vi "Main.vi"() -> ()   [LabVIEW 2013]
uses:
  <vilib>/Utility/miscctls.llb/LVFontTypeDef.ctl
panel:
  in  "SetCurrent":dbl min=0.0 max=72.0 step=0.1 format="%#.1g"
  in  "SetVoltage":dbl min=0.0 max=30.0 step=0.1 format="%#.1g"
  in  "SetCurrentB":bool
  in  "SetVoltageB":bool
  in  "Comm. current %":dbl=0.5 caption="%" min=0.0 max=100.0 step=0.5
  in  "Common curr. dec":bool
  in  "Common curr. inc":bool
  out "Дата":string
  out "Время":string
  in  "SetCurrentAll":bool
  in  "SetVoltageAll":bool
  in  "ConnectAll":bool
  in  "DisconnectAll":bool
  in  "Set Output ON All":bool caption="ВЫХОДЫ ИСТОЧНИКОВ"
  in  "Comm. voltage %":dbl caption="%" min=0.0 max=100.0 step=0.5
  in  "Common volt. dec":bool
  in  "Common volt. inc":bool
  in  "ReadFromFile":bool
  in  "WriteToFile":bool
  in  "SetOutputOffB":bool
  in  "SetOutputOnB":bool
  in  "ConnectChannel":bool
  in  "DisconnectChannel":bool
  in  "Имя":string="55"
  in  "DeleteChannel":bool
  in  "IP":string="172.16.21.19"
  in  "AddChannel":bool
  out "CURRENTSET":dbl[](array[numeric])
  in  "CurrentModulationOn":bool
  in  "Amp":dbl
  in  "CurrentModulationB":bool
  out "NAME":string[](array[string])
  out "ADRESS":string[](array[string])
  out "VIRef":refnum<vi>[](array[refnum])
  in  "Quit":bool
  in  "List of channels":i32(listbox)
  # "ВСЕ ИСТОЧНИКИ"
  # "1 ИСТОЧНИК"
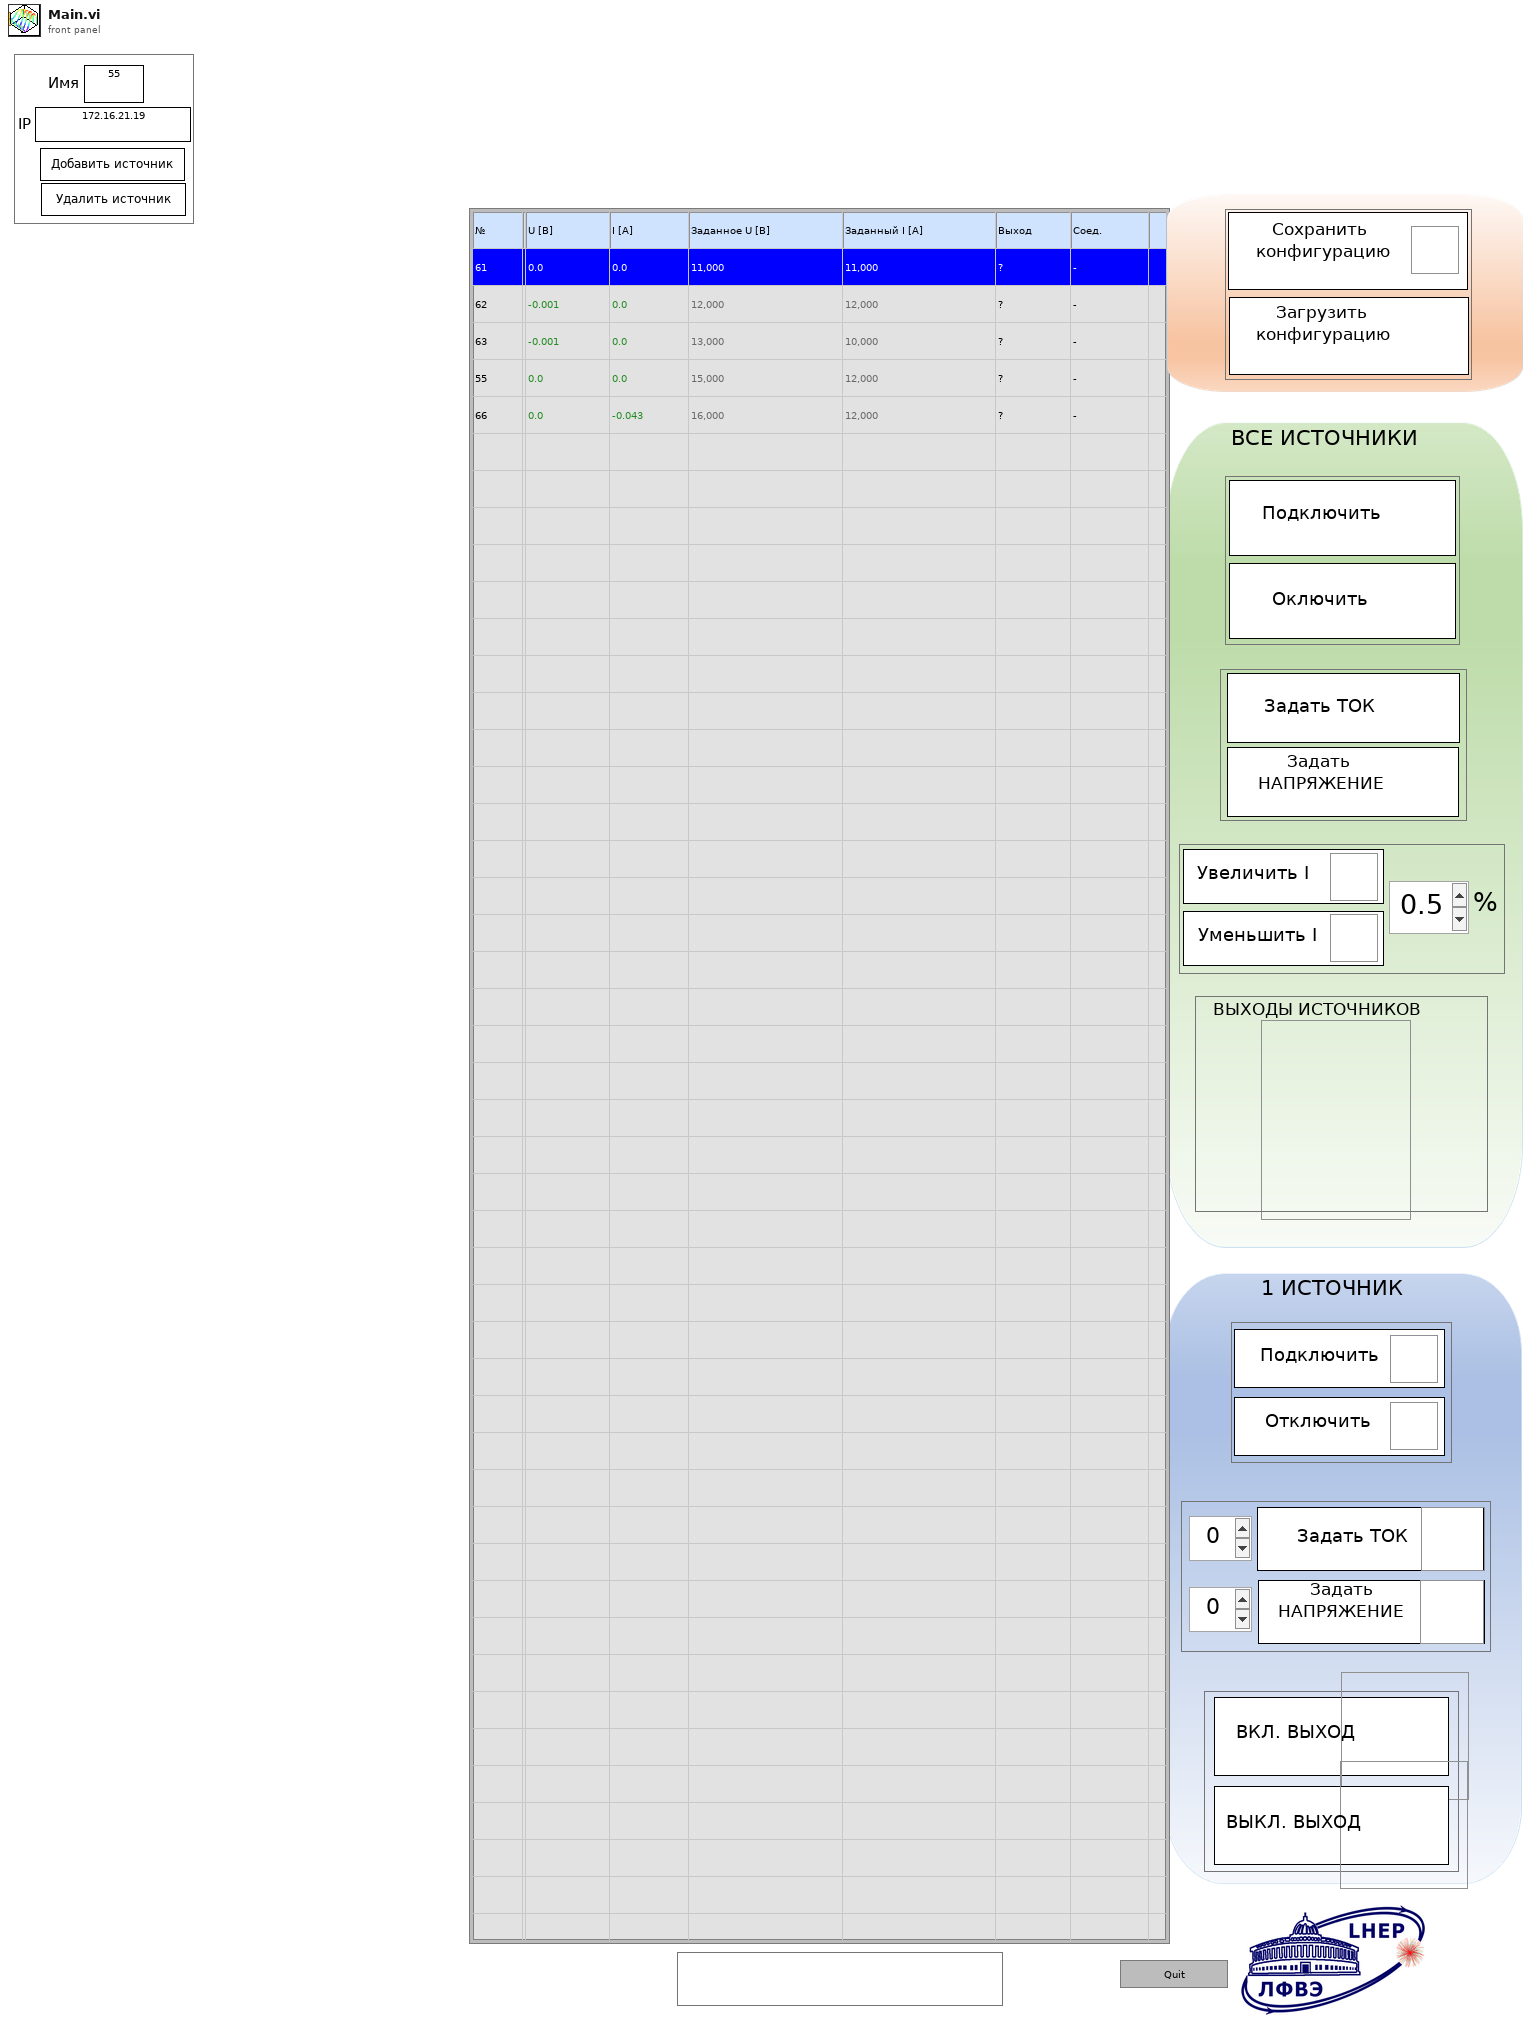
[diagram p1: front panel]
types:
  T1 = typedef "LVFontTypeDef.ctl" = cluster{"Font Name":string, "Size":u16, "Bold":bool, "Italic":bool, "Underline":bool, "Strikeout":bool, "Color":u32}
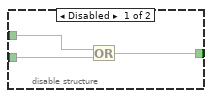
[diagram p3: hidden frame]
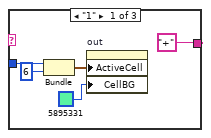
[diagram p4: hidden frame]
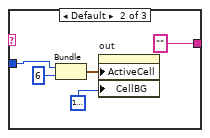
[diagram p5: hidden frame]
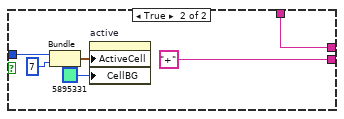
[diagram p6: hidden frame]
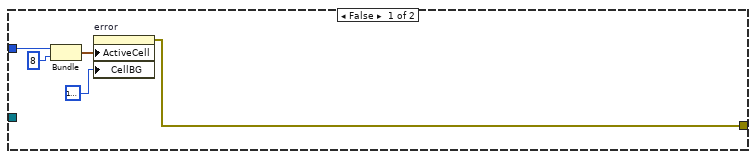
[diagram p7: hidden frame]
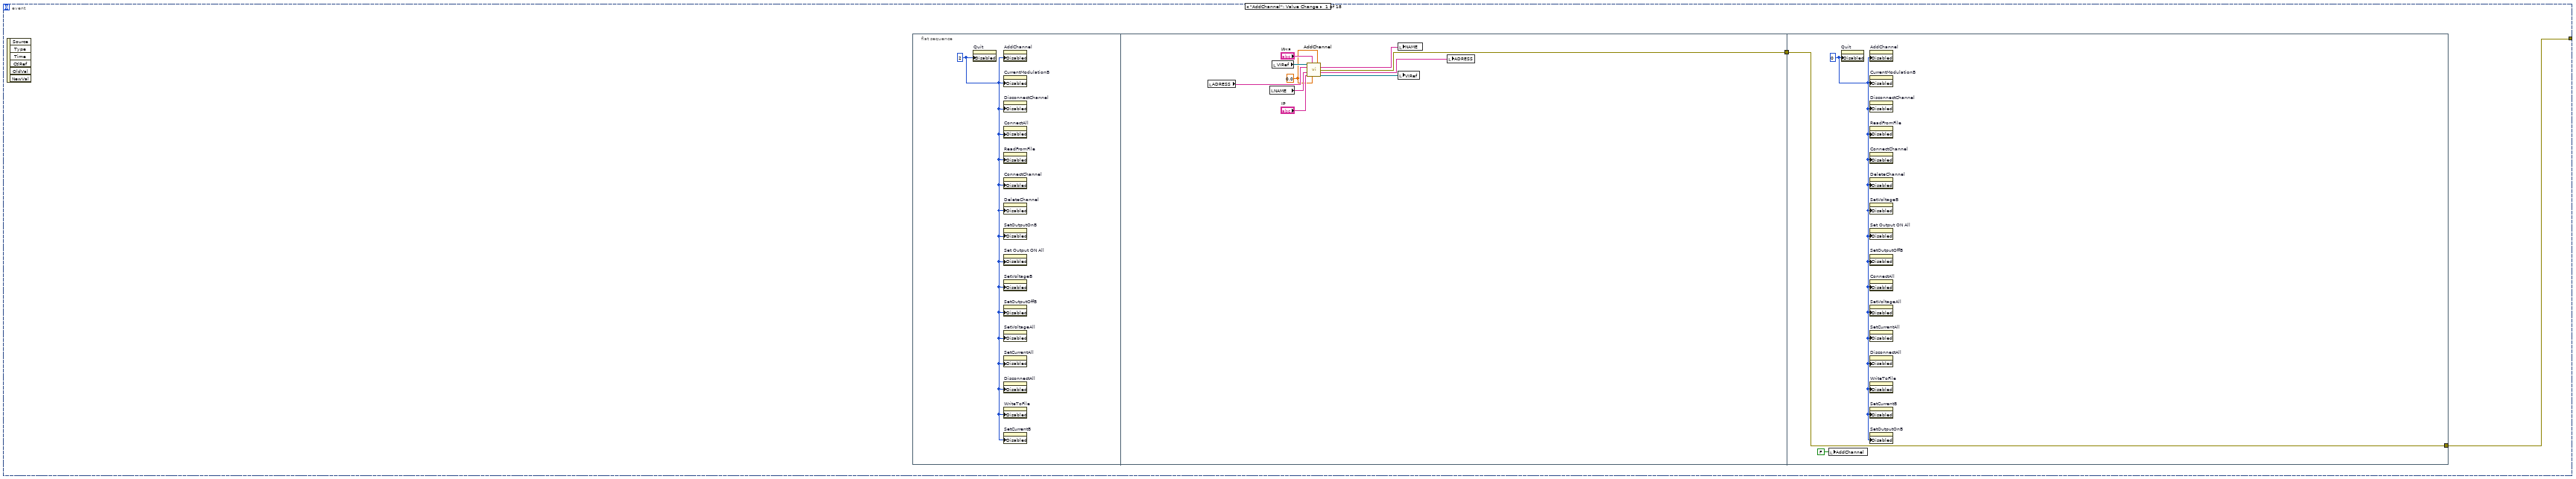
[diagram p8: hidden frame]
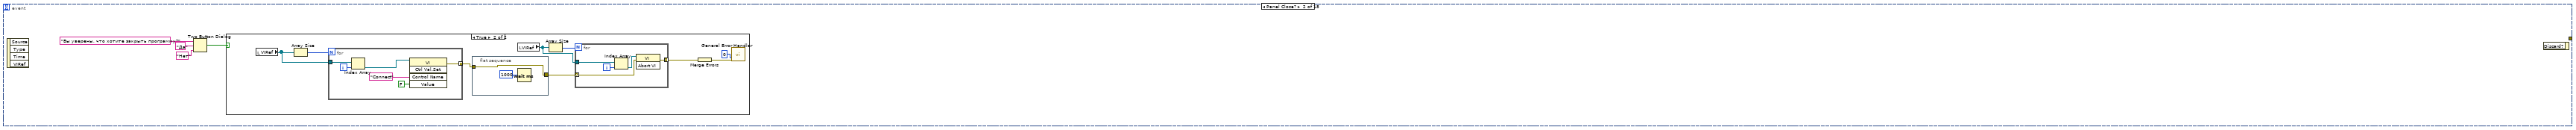
[diagram p9: hidden frame]
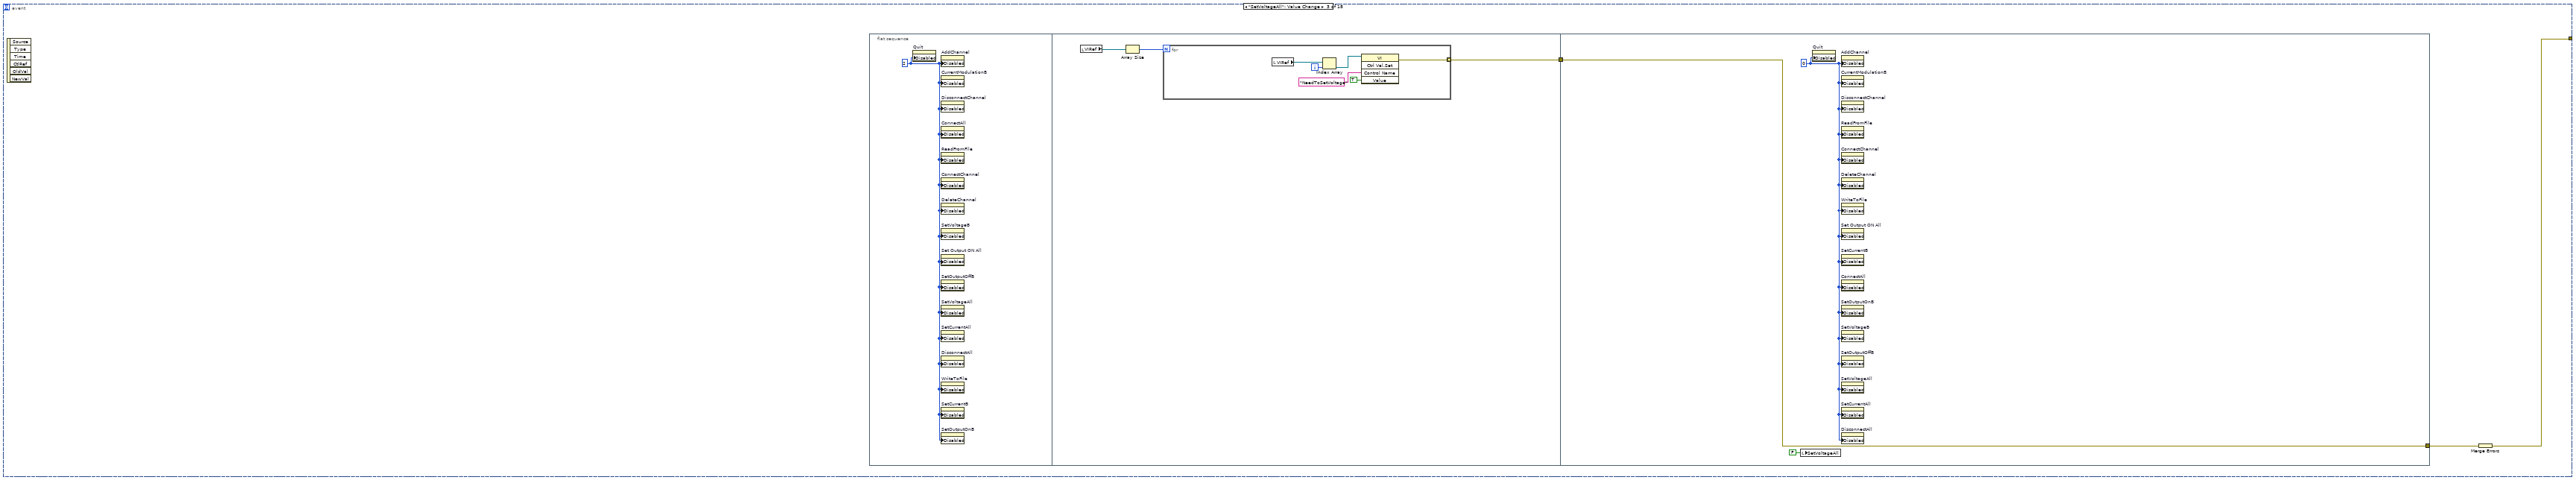
[diagram p11: hidden frame]
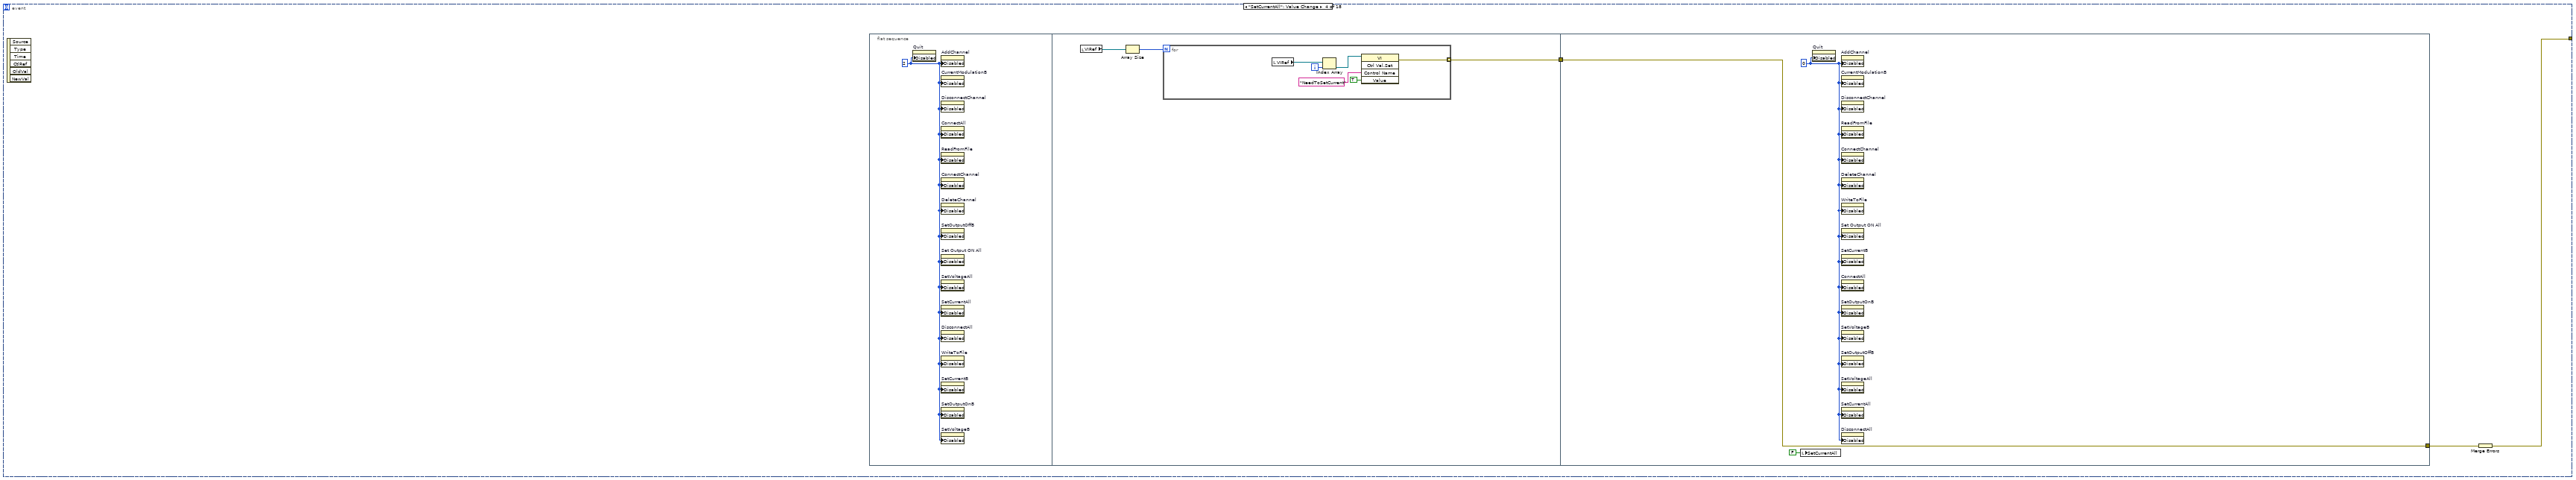
[diagram p12: hidden frame]
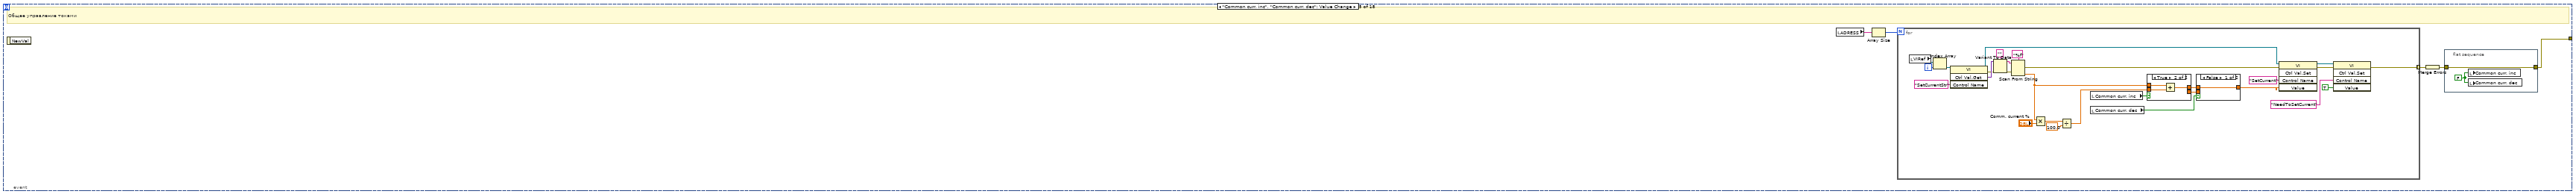
[diagram p13: hidden frame]
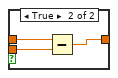
[diagram p14: hidden frame]
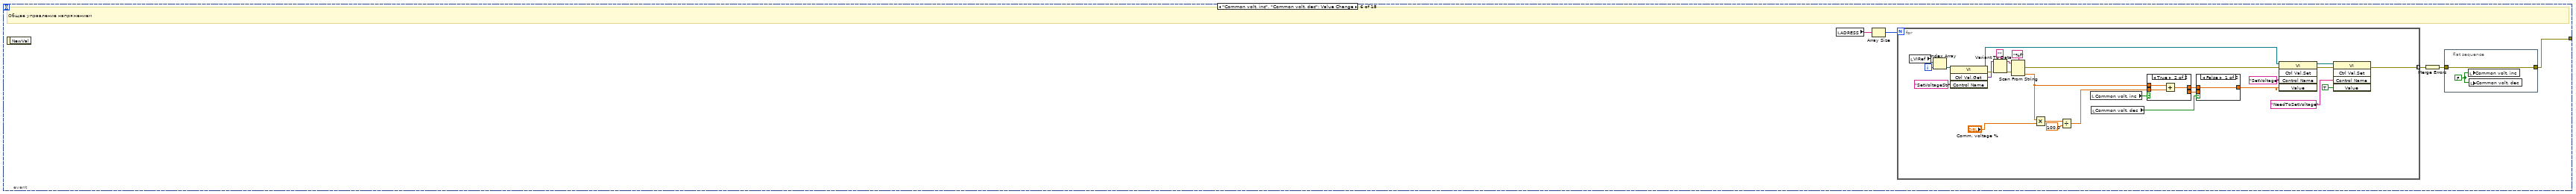
[diagram p16: hidden frame]
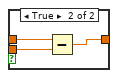
[diagram p17: hidden frame]
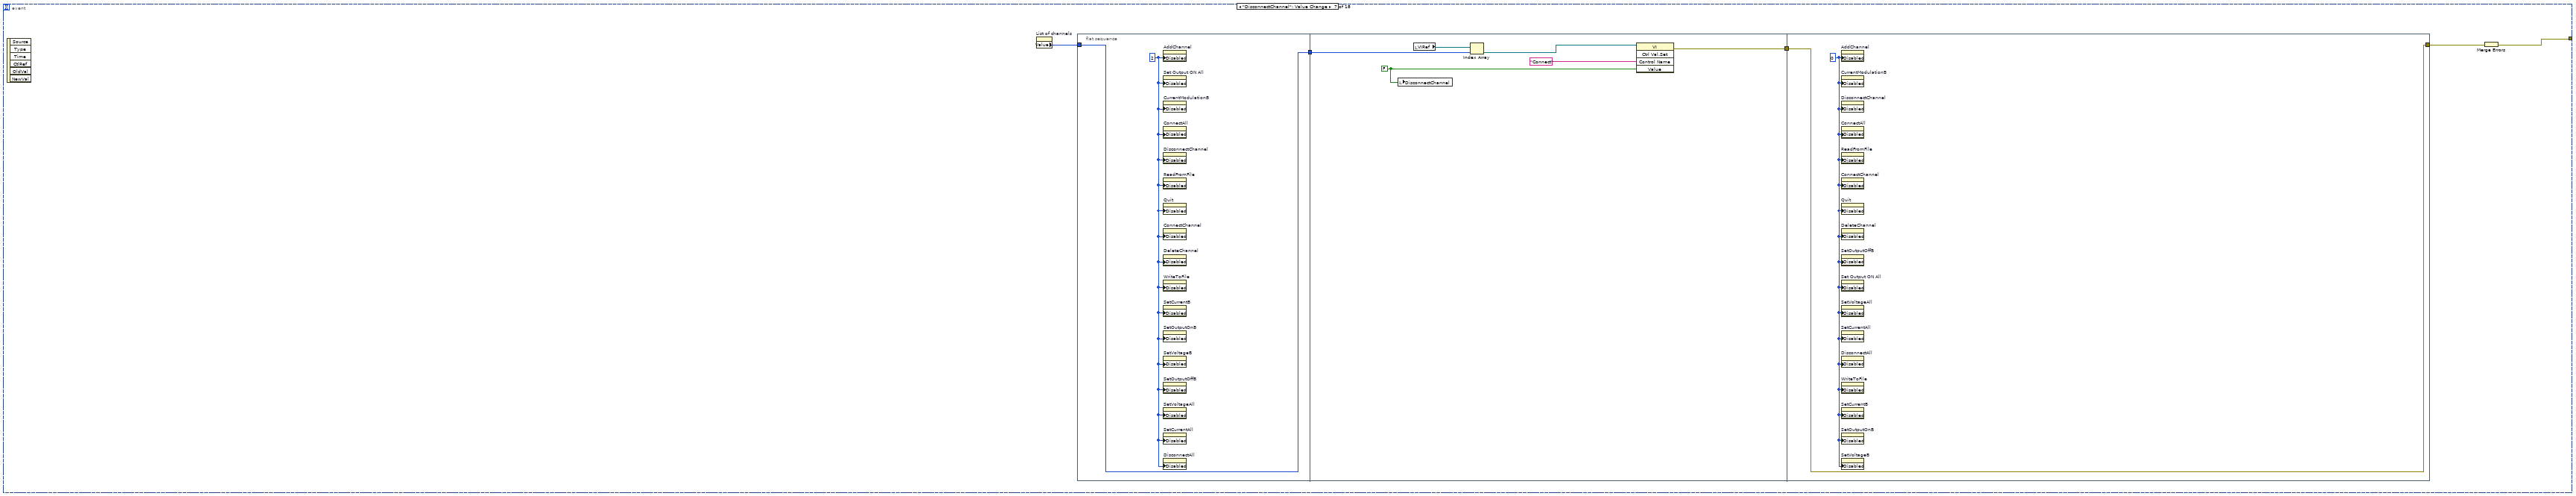
[diagram p19: hidden frame]
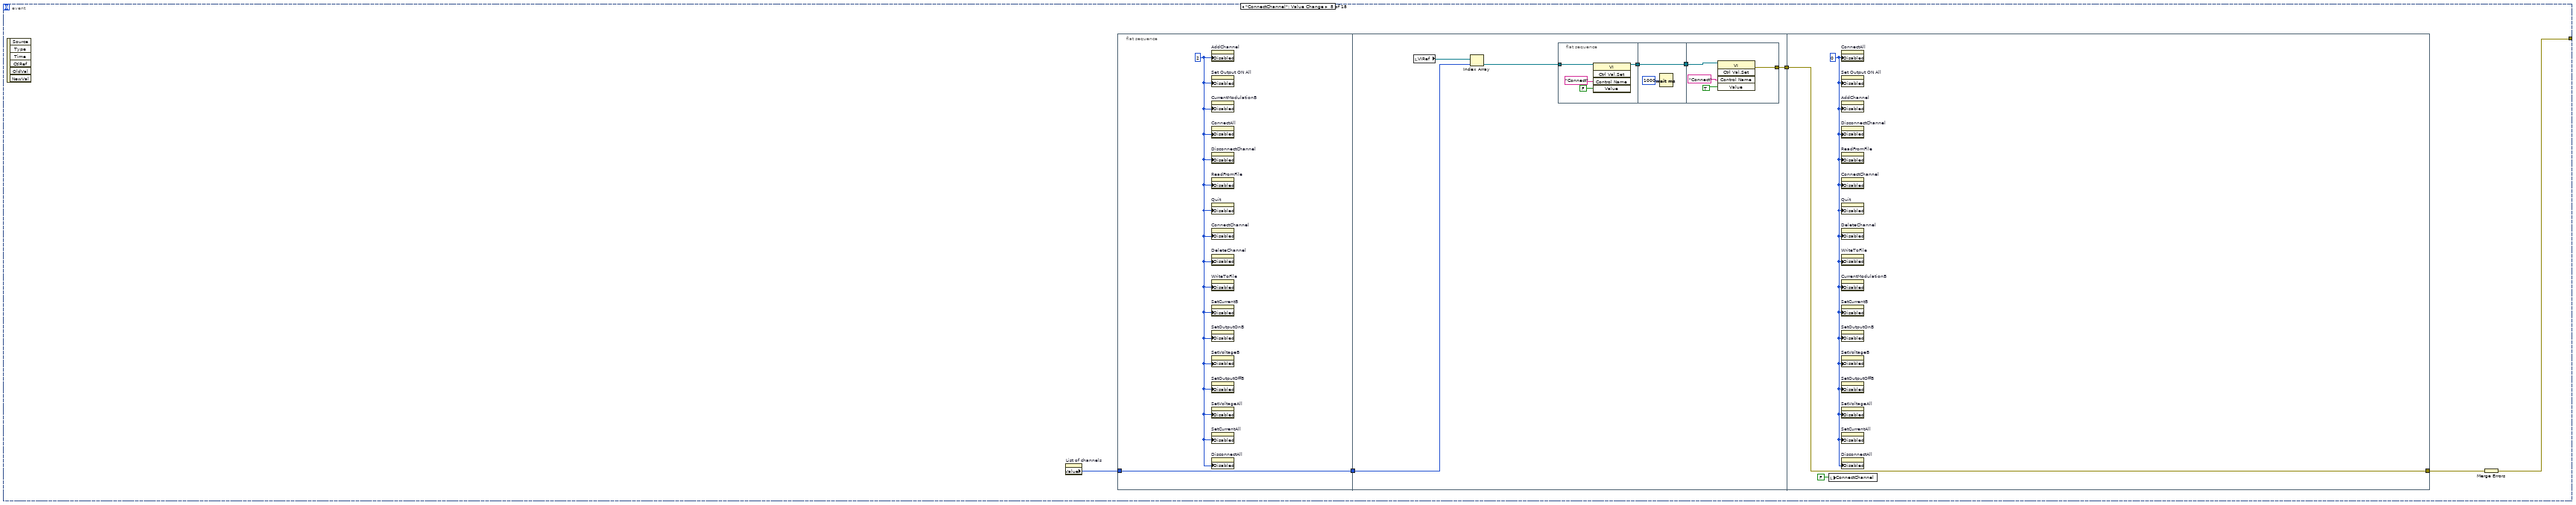
[diagram p20: hidden frame]
diagram:
  w18 = u8 0 ("Disabled")
  w20 = FALSE ("SetOutputOnB")
  w21 = FALSE ("OK Button")
  n1 = event shown="[0] \"Quit\": Value Change" {
    selector: _ -> [_]
    dyn-events: _ -> [_]
    timeout: _ -> [_]
    event "Quit": Value Change {
      n2 = event-data() -> ()  [unwired: 1 in, 5 out]
      n3 = Stop(stop? (T)=TRUE) -> ()
    }
  }
  n4 = while {
    stop <- FALSE stop-if-true
    n5 = Get Date/Time String(want seconds? (F)=TRUE) -> (date string=→"Дата":string, time string=→"Время":string)  [unwired: 2 in]
    n6 = Wait Until Next ms Multiple(millisecond multiple=u16 1000) -> ()  [unwired: 1 out]
  }
  n7 = while {
    stop <- FALSE stop-if-true
    n8 = event shown="[11] \"SetOutputOnB\": Value Change" {
      selector: _ -> [_ _ _ _ _ _ _ _ _ _ _ _ _ _ _ _ _ _]
      dyn-events: _ -> [_ _ _ _ _ _ _ _ _ _ _ _ _ _ _ _ _ _]
      timeout: _ -> [_ _ _ _ _ _ _ _ _ _ _ _ _ _ _ _ _ _]
      tunnel: [w35 _ w77 w93 w109 w153 w197 w212 w238 w254 w270 w287 w308 w331 w349 w400 w474 w497] -> w32
      event "AddChannel": Value Change {
        n9 = event-data() -> ()  [unwired: 7 out]
        n10 = flat-sequence {
          tunnel: [w38] -> w36
          tunnel: [w48] -> w35
          tunnel: w36 -> [w48]
          frame #0 {
            w37 = u8 2 ("Disabled")
            n11 = property on="Quit" class="Bool (strict)"("Disabled"=w37) -> ()  [unwired: 2 in, 2 out]
            n12 = property on="AddChannel" class="Bool (strict)"("Disabled"=w37) -> ()  [unwired: 2 in, 2 out]
            n13 = property on="CurrentModulationB" class="Bool (strict)"("Disabled"=w37) -> ()  [unwired: 2 in, 2 out]
            n14 = property on="DisconnectChannel" class="Bool (strict)"("Disabled"=w37) -> ()  [unwired: 2 in, 2 out]
            n15 = property on="ConnectAll" class="Bool (strict)"("Disabled"=w37) -> ()  [unwired: 2 in, 2 out]
            n16 = property on="ReadFromFile" class="Bool (strict)"("Disabled"=w37) -> ()  [unwired: 2 in, 2 out]
            n17 = property on="ConnectChannel" class="Bool (strict)"("Disabled"=w37) -> ()  [unwired: 2 in, 2 out]
            n18 = property on="DeleteChannel" class="Bool (strict)"("Disabled"=w37) -> ()  [unwired: 2 in, 2 out]
            n19 = property on="SetOutputOnB" class="Bool (strict)"("Disabled"=w37) -> ()  [unwired: 2 in, 2 out]
            n20 = property on="Set Output ON All" class="Bool (strict)"("Disabled"=w37) -> ()  [unwired: 2 in, 2 out]
            n21 = property on="SetVoltageB" class="Bool (strict)"("Disabled"=w37) -> ()  [unwired: 2 in, 2 out]
            n22 = property on="SetOutputOffB" class="Bool (strict)"("Disabled"=w37) -> ()  [unwired: 2 in, 2 out]
            n23 = property on="SetVoltageAll" class="Bool (strict)"("Disabled"=w37) -> ()  [unwired: 2 in, 2 out]
            n24 = property on="SetCurrentAll" class="Bool (strict)"("Disabled"=w37) -> ()  [unwired: 2 in, 2 out]
            n25 = property on="DisconnectAll" class="Bool (strict)"("Disabled"=w37) -> ()  [unwired: 2 in, 2 out]
            n26 = property on="WriteToFile" class="Bool (strict)"("Disabled"=w37) -> ()  [unwired: 2 in, 2 out]
            n27 = property on="SetCurrentB" class="Bool (strict)"("Disabled"=w37) -> ()  [unwired: 2 in, 2 out]
          }
          frame #1 {
            w39 = 0.0 ("SetVoltage")
            n28 = local read "ADRESS"() -> (w45:string[])
            n29 = local read "NAME"() -> (w44:string[])
            n30 = local read "VIRef"() -> (w43:refnum<vi>[])
            n31 = call "AddChannel.vi"("VIRef"=w43, "Name"="Имя", "SetCurrent"=w39, "ADRESS"=w45, "NAME"=w44, "Address"="IP", "SetVoltage"=w39) -> ("NAMEOut"=w40:string[], "error out"=w38:errorcluster, "ADRESSOut"=w41:string[], "VIRefOut"=w42:refnum<vi>[])  [unwired: 1 in, 4 out]
            n32 = local write "NAME"(w40) -> ()
            n33 = local write "VIRef"(w42) -> ()
            n34 = local write "ADRESS"(w41) -> ()
          }
          frame #2 {
            w49 = u8 0 ("Disabled")
            n35 = local write "AddChannel"(FALSE ("AddChannel")) -> ()
            n36 = property on="Quit" class="Bool (strict)"("Disabled"=w49) -> ()  [unwired: 2 in, 2 out]
            n37 = property on="AddChannel" class="Bool (strict)"("Disabled"=w49) -> ()  [unwired: 2 in, 2 out]
            n38 = property on="CurrentModulationB" class="Bool (strict)"("Disabled"=w49) -> ()  [unwired: 2 in, 2 out]
            n39 = property on="DisconnectChannel" class="Bool (strict)"("Disabled"=w49) -> ()  [unwired: 2 in, 2 out]
            n40 = property on="ReadFromFile" class="Bool (strict)"("Disabled"=w49) -> ()  [unwired: 2 in, 2 out]
            n41 = property on="ConnectChannel" class="Bool (strict)"("Disabled"=w49) -> ()  [unwired: 2 in, 2 out]
            n42 = property on="DeleteChannel" class="Bool (strict)"("Disabled"=w49) -> ()  [unwired: 2 in, 2 out]
            n43 = property on="SetVoltageB" class="Bool (strict)"("Disabled"=w49) -> ()  [unwired: 2 in, 2 out]
            n44 = property on="Set Output ON All" class="Bool (strict)"("Disabled"=w49) -> ()  [unwired: 2 in, 2 out]
            n45 = property on="SetOutputOffB" class="Bool (strict)"("Disabled"=w49) -> ()  [unwired: 2 in, 2 out]
            n46 = property on="ConnectAll" class="Bool (strict)"("Disabled"=w49) -> ()  [unwired: 2 in, 2 out]
            n47 = property on="SetVoltageAll" class="Bool (strict)"("Disabled"=w49) -> ()  [unwired: 2 in, 2 out]
            n48 = property on="SetCurrentAll" class="Bool (strict)"("Disabled"=w49) -> ()  [unwired: 2 in, 2 out]
            n49 = property on="DisconnectAll" class="Bool (strict)"("Disabled"=w49) -> ()  [unwired: 2 in, 2 out]
            n50 = property on="WriteToFile" class="Bool (strict)"("Disabled"=w49) -> ()  [unwired: 2 in, 2 out]
            n51 = property on="SetCurrentB" class="Bool (strict)"("Disabled"=w49) -> ()  [unwired: 2 in, 2 out]
            n52 = property on="SetOutputOnB" class="Bool (strict)"("Disabled"=w49) -> ()  [unwired: 2 in, 2 out]
          }
        }
      }
      event Panel Close? {
        n53 = event-data() -> ()  [unwired: 5 out]
        n54 = Two Button Dialog(message="Вы уверены, что хотите закрыть программу?", 1:"Нет" ("F button name (\"Cancel\")"), 2:"Да" ("T button name (\"OK\")")) -> (T button?=w54:bool)
        n55 = case shown="True" w54 {
          frame False {
          }
          frame True {
            n56 = local read "VIRef"() -> (w56:refnum<vi>[])
            n57 = Array Size(array=w56) -> (size(s)=w55:i32)
            n58 = for {
              N: w55 -> [_]
              tunnel: w56 -> [w73]
              tunnel: [w71] -> w63 mode=indexing
              i -> [w74]
              n59 = Index Array(array=w73, index=w74) -> (element=w72:refnum<vi>)
              n60 = invoke class="VI" method="Ctrl Val.Set"(reference=w72, "Control Name"="Connect", "Value"=FALSE) -> (error out=w71:errorcluster)  [unwired: 2 in, 4 out]
            }
            n61 = flat-sequence {
              tunnel: [w65] -> w62
              tunnel: w63 -> [w65]
              frame #0 {
                n62 = Wait (ms)(milliseconds to wait=u32 1000) -> ()  [unwired: 1 out]
              }
            }
            n63 = local read "VIRef"() -> (w57:refnum<vi>[])
            n64 = Array Size(array=w57) -> (size(s)=w58:i32)
            n65 = for {
              N: w58 -> [_]
              tunnel: w57 -> [w69]
              tunnel: [w67] -> w59 mode=indexing
              tunnel: w62 -> [w66] mode=indexing
              i -> [w70]
              n66 = Index Array(array=w69, index=w70) -> (element=w68:refnum<vi>)
              n67 = invoke class="VI" method="Abort VI"(reference=w68, error in=w66) -> (error out=w67:errorcluster)  [unwired: 1 in, 2 out]
            }
            n68 = Merge Errors(w59) -> (w60:errorcluster)
            n69 = call <vilib>:"General Error Handler.vi"("type of dialog (OK msg:1)"=u32 0 ("milliseconds to wait"), "error in (no error)"=w60) -> ()  [unwired: 9 in, 5 out]
          }
        }
        n70 = event-data() -> ()  [unwired: 2 in, 1 out]
      }
      event "SetVoltageAll": Value Change {
        n71 = event-data() -> ()  [unwired: 7 out]
        n72 = flat-sequence {
          tunnel: [w81] -> w79
          tunnel: [w90] -> w78
          tunnel: w79 -> [w90]
          frame #0 {
            w80 = u8 2 ("Disabled")
            n73 = property on="Quit" class="Bool (strict)"("Disabled"=w80) -> ()  [unwired: 2 in, 2 out]
            n74 = property on="AddChannel" class="Bool (strict)"("Disabled"=w80) -> ()  [unwired: 2 in, 2 out]
            n75 = property on="CurrentModulationB" class="Bool (strict)"("Disabled"=w80) -> ()  [unwired: 2 in, 2 out]
            n76 = property on="DisconnectChannel" class="Bool (strict)"("Disabled"=w80) -> ()  [unwired: 2 in, 2 out]
            n77 = property on="ConnectAll" class="Bool (strict)"("Disabled"=w80) -> ()  [unwired: 2 in, 2 out]
            n78 = property on="ReadFromFile" class="Bool (strict)"("Disabled"=w80) -> ()  [unwired: 2 in, 2 out]
            n79 = property on="ConnectChannel" class="Bool (strict)"("Disabled"=w80) -> ()  [unwired: 2 in, 2 out]
            n80 = property on="DeleteChannel" class="Bool (strict)"("Disabled"=w80) -> ()  [unwired: 2 in, 2 out]
            n81 = property on="SetVoltageB" class="Bool (strict)"("Disabled"=w80) -> ()  [unwired: 2 in, 2 out]
            n82 = property on="Set Output ON All" class="Bool (strict)"("Disabled"=w80) -> ()  [unwired: 2 in, 2 out]
            n83 = property on="SetOutputOffB" class="Bool (strict)"("Disabled"=w80) -> ()  [unwired: 2 in, 2 out]
            n84 = property on="SetVoltageAll" class="Bool (strict)"("Disabled"=w80) -> ()  [unwired: 2 in, 2 out]
            n85 = property on="SetCurrentAll" class="Bool (strict)"("Disabled"=w80) -> ()  [unwired: 2 in, 2 out]
            n86 = property on="DisconnectAll" class="Bool (strict)"("Disabled"=w80) -> ()  [unwired: 2 in, 2 out]
            n87 = property on="WriteToFile" class="Bool (strict)"("Disabled"=w80) -> ()  [unwired: 2 in, 2 out]
            n88 = property on="SetCurrentB" class="Bool (strict)"("Disabled"=w80) -> ()  [unwired: 2 in, 2 out]
            n89 = property on="SetOutputOnB" class="Bool (strict)"("Disabled"=w80) -> ()  [unwired: 2 in, 2 out]
          }
          frame #1 {
            n90 = local read "VIRef"() -> (w83:refnum<vi>[])
            n91 = Array Size(array=w83) -> (size(s)=w82:i32)
            n92 = for {
              N: w82 -> [_]
              tunnel: [w84] -> w81 mode=indexing
              i -> [w86]
              n93 = local read "VIRef"() -> (w89:refnum<vi>[])
              n94 = Index Array(array=w89, index=w86) -> (element=w85:refnum<vi>)
              n95 = invoke class="VI" method="Ctrl Val.Set"(reference=w85, "Control Name"="NeedToSetVoltage", "Value"=TRUE ("ConnectChannel")) -> (error out=w84:errorcluster)  [unwired: 2 in, 4 out]
            }
          }
          frame #2 {
            w91 = u8 0 ("Disabled")
            n96 = local write "SetVoltageAll"(FALSE ("SetVoltageAll")) -> ()
            n97 = property on="Quit" class="Bool (strict)"("Disabled"=w91) -> ()  [unwired: 2 in, 2 out]
            n98 = property on="AddChannel" class="Bool (strict)"("Disabled"=w91) -> ()  [unwired: 2 in, 2 out]
            n99 = property on="CurrentModulationB" class="Bool (strict)"("Disabled"=w91) -> ()  [unwired: 2 in, 2 out]
            n100 = property on="DisconnectChannel" class="Bool (strict)"("Disabled"=w91) -> ()  [unwired: 2 in, 2 out]
            n101 = property on="ReadFromFile" class="Bool (strict)"("Disabled"=w91) -> ()  [unwired: 2 in, 2 out]
            n102 = property on="ConnectChannel" class="Bool (strict)"("Disabled"=w91) -> ()  [unwired: 2 in, 2 out]
            n103 = property on="DeleteChannel" class="Bool (strict)"("Disabled"=w91) -> ()  [unwired: 2 in, 2 out]
            n104 = property on="WriteToFile" class="Bool (strict)"("Disabled"=w91) -> ()  [unwired: 2 in, 2 out]
            n105 = property on="Set Output ON All" class="Bool (strict)"("Disabled"=w91) -> ()  [unwired: 2 in, 2 out]
            n106 = property on="SetCurrentB" class="Bool (strict)"("Disabled"=w91) -> ()  [unwired: 2 in, 2 out]
            n107 = property on="ConnectAll" class="Bool (strict)"("Disabled"=w91) -> ()  [unwired: 2 in, 2 out]
            n108 = property on="SetOutputOnB" class="Bool (strict)"("Disabled"=w91) -> ()  [unwired: 2 in, 2 out]
            n109 = property on="SetVoltageB" class="Bool (strict)"("Disabled"=w91) -> ()  [unwired: 2 in, 2 out]
            n110 = property on="SetOutputOffB" class="Bool (strict)"("Disabled"=w91) -> ()  [unwired: 2 in, 2 out]
            n111 = property on="SetVoltageAll" class="Bool (strict)"("Disabled"=w91) -> ()  [unwired: 2 in, 2 out]
            n112 = property on="SetCurrentAll" class="Bool (strict)"("Disabled"=w91) -> ()  [unwired: 2 in, 2 out]
            n113 = property on="DisconnectAll" class="Bool (strict)"("Disabled"=w91) -> ()  [unwired: 2 in, 2 out]
          }
        }
        n114 = Merge Errors(w78) -> (w77:errorcluster)
      }
      event "SetCurrentAll": Value Change {
        n115 = event-data() -> ()  [unwired: 7 out]
        n116 = flat-sequence {
          tunnel: [w97] -> w95
          tunnel: [w106] -> w94
          tunnel: w95 -> [w106]
          frame #0 {
            w96 = u8 2 ("Disabled")
            n117 = property on="Quit" class="Bool (strict)"("Disabled"=w96) -> ()  [unwired: 2 in, 2 out]
            n118 = property on="AddChannel" class="Bool (strict)"("Disabled"=w96) -> ()  [unwired: 2 in, 2 out]
            n119 = property on="CurrentModulationB" class="Bool (strict)"("Disabled"=w96) -> ()  [unwired: 2 in, 2 out]
            n120 = property on="DisconnectChannel" class="Bool (strict)"("Disabled"=w96) -> ()  [unwired: 2 in, 2 out]
            n121 = property on="ConnectAll" class="Bool (strict)"("Disabled"=w96) -> ()  [unwired: 2 in, 2 out]
            n122 = property on="ReadFromFile" class="Bool (strict)"("Disabled"=w96) -> ()  [unwired: 2 in, 2 out]
            n123 = property on="ConnectChannel" class="Bool (strict)"("Disabled"=w96) -> ()  [unwired: 2 in, 2 out]
            n124 = property on="DeleteChannel" class="Bool (strict)"("Disabled"=w96) -> ()  [unwired: 2 in, 2 out]
            n125 = property on="SetOutputOffB" class="Bool (strict)"("Disabled"=w96) -> ()  [unwired: 2 in, 2 out]
            n126 = property on="Set Output ON All" class="Bool (strict)"("Disabled"=w96) -> ()  [unwired: 2 in, 2 out]
            n127 = property on="SetVoltageAll" class="Bool (strict)"("Disabled"=w96) -> ()  [unwired: 2 in, 2 out]
            n128 = property on="SetCurrentAll" class="Bool (strict)"("Disabled"=w96) -> ()  [unwired: 2 in, 2 out]
            n129 = property on="DisconnectAll" class="Bool (strict)"("Disabled"=w96) -> ()  [unwired: 2 in, 2 out]
            n130 = property on="WriteToFile" class="Bool (strict)"("Disabled"=w96) -> ()  [unwired: 2 in, 2 out]
            n131 = property on="SetCurrentB" class="Bool (strict)"("Disabled"=w96) -> ()  [unwired: 2 in, 2 out]
            n132 = property on="SetOutputOnB" class="Bool (strict)"("Disabled"=w96) -> ()  [unwired: 2 in, 2 out]
            n133 = property on="SetVoltageB" class="Bool (strict)"("Disabled"=w96) -> ()  [unwired: 2 in, 2 out]
          }
          frame #1 {
            n134 = local read "VIRef"() -> (w99:refnum<vi>[])
            n135 = Array Size(array=w99) -> (size(s)=w98:i32)
            n136 = for {
              N: w98 -> [_]
              tunnel: [w100] -> w97 mode=indexing
              i -> [w102]
              n137 = local read "VIRef"() -> (w105:refnum<vi>[])
              n138 = Index Array(array=w105, index=w102) -> (element=w101:refnum<vi>)
              n139 = invoke class="VI" method="Ctrl Val.Set"(reference=w101, "Control Name"="NeedToSetCurrent", "Value"=TRUE ("ConnectChannel")) -> (error out=w100:errorcluster)  [unwired: 2 in, 4 out]
            }
          }
          frame #2 {
            w107 = u8 0 ("Disabled")
            n140 = local write "SetCurrentAll"(FALSE ("SetVoltageAll")) -> ()
            n141 = property on="Quit" class="Bool (strict)"("Disabled"=w107) -> ()  [unwired: 2 in, 2 out]
            n142 = property on="AddChannel" class="Bool (strict)"("Disabled"=w107) -> ()  [unwired: 2 in, 2 out]
            n143 = property on="CurrentModulationB" class="Bool (strict)"("Disabled"=w107) -> ()  [unwired: 2 in, 2 out]
            n144 = property on="DisconnectChannel" class="Bool (strict)"("Disabled"=w107) -> ()  [unwired: 2 in, 2 out]
            n145 = property on="ReadFromFile" class="Bool (strict)"("Disabled"=w107) -> ()  [unwired: 2 in, 2 out]
            n146 = property on="ConnectChannel" class="Bool (strict)"("Disabled"=w107) -> ()  [unwired: 2 in, 2 out]
            n147 = property on="DeleteChannel" class="Bool (strict)"("Disabled"=w107) -> ()  [unwired: 2 in, 2 out]
            n148 = property on="WriteToFile" class="Bool (strict)"("Disabled"=w107) -> ()  [unwired: 2 in, 2 out]
            n149 = property on="Set Output ON All" class="Bool (strict)"("Disabled"=w107) -> ()  [unwired: 2 in, 2 out]
            n150 = property on="SetCurrentB" class="Bool (strict)"("Disabled"=w107) -> ()  [unwired: 2 in, 2 out]
            n151 = property on="ConnectAll" class="Bool (strict)"("Disabled"=w107) -> ()  [unwired: 2 in, 2 out]
            n152 = property on="SetOutputOnB" class="Bool (strict)"("Disabled"=w107) -> ()  [unwired: 2 in, 2 out]
            n153 = property on="SetVoltageB" class="Bool (strict)"("Disabled"=w107) -> ()  [unwired: 2 in, 2 out]
            n154 = property on="SetOutputOffB" class="Bool (strict)"("Disabled"=w107) -> ()  [unwired: 2 in, 2 out]
            n155 = property on="SetVoltageAll" class="Bool (strict)"("Disabled"=w107) -> ()  [unwired: 2 in, 2 out]
            n156 = property on="SetCurrentAll" class="Bool (strict)"("Disabled"=w107) -> ()  [unwired: 2 in, 2 out]
            n157 = property on="DisconnectAll" class="Bool (strict)"("Disabled"=w107) -> ()  [unwired: 2 in, 2 out]
          }
        }
        n158 = Merge Errors(w94) -> (w93:errorcluster)
      }
      event "Common curr. inc", "Common curr. dec": Value Change {
        # "Общее управление токами"
        n159 = event-data() -> ()  [unwired: 2 out]
        n160 = local read "ADRESS"() -> (w112:string[])
        n161 = Array Size(array=w112) -> (size(s)=w113:i32)
        n162 = for {
          N: w113 -> [_]
          tunnel: [w122] -> w111 mode=indexing
          i -> [w140]
          n163 = local read "VIRef"() -> (w143:refnum<vi>[])
          n164 = Index Array(array=w143, index=w140) -> (element=w130:refnum<vi>)
          n165 = invoke class="VI" method="Ctrl Val.Get"(reference=w130, "Control Name"="SetCurrentStr") -> (reference out=w124:refnum<vi>, error out=w138:errorcluster, "Get Control Value Variant"=w142:variant)  [unwired: 2 in, 1 out]
          n166 = Variant To Data(error in=w138, type="" ("Control Name"), Variant=w142) -> (data=w137:string, error out=w136:errorcluster)
          n167 = Scan From String(format string="%f", input string=w137, error in=w136) -> (error out=w123:errorcluster, output 1=w121:dbl)  [unwired: 2 in, 2 out]
          n168 = Multiply(x=w121, y="Comm. current %") -> (x*y=w132:dbl)
          n169 = Divide(x=w132, y=100.0) -> (x/y=w134:dbl)
          n170 = local read "Common curr. inc"() -> (w120:bool)
          n171 = local read "Common curr. dec"() -> (w118:bool)
          n172 = case shown="True" w120 {
            tunnel: w134 -> [w148 w152]
            tunnel: w121 -> [w149 w151]
            tunnel: [w149 w150] -> w119
            tunnel: [w148 _] -> w117
            frame False {
            }
            frame True {
              n173 = Add(x=w151, y=w152) -> (x+y=w150:dbl)
            }
          }
          n174 = case shown="False" w118 {
            tunnel: w119 -> [w144 w147]
            tunnel: [w144 w146] -> w116
            tunnel: w117 -> [_ w145]
            frame False {
            }
            frame True {
              n175 = Subtract(x=w147, y=w145) -> (x-y=w146:dbl)
            }
          }
          n176 = invoke class="VI" method="Ctrl Val.Set"(reference=w124, error in=w123, "Control Name"="SetCurrent", "Value"=w116) -> (reference out=w126:refnum<vi>, error out=w125:errorcluster)  [unwired: 1 in, 3 out]
          n177 = invoke class="VI" method="Ctrl Val.Set"(reference=w126, error in=w125, "Control Name"="NeedToSetCurrent", "Value"=TRUE ("ConnectChannel")) -> (error out=w122:errorcluster)  [unwired: 1 in, 4 out]
        }
        n178 = Merge Errors(w111) -> (w110:errorcluster)
        n179 = flat-sequence {
          tunnel: w110 -> [w115]
          tunnel: [w115] -> w109
          frame #0 {
            w114 = FALSE ("ConnectChannel")
            n180 = local write "Common curr. inc"(w114) -> ()
            n181 = local write "Common curr. dec"(w114) -> ()
          }
        }
      }
      event "Common volt. inc", "Common volt. dec": Value Change {
        # "Общее управление напряжением"
        n182 = event-data() -> ()  [unwired: 2 out]
        n183 = local read "ADRESS"() -> (w156:string[])
        n184 = Array Size(array=w156) -> (size(s)=w157:i32)
        n185 = for {
          N: w157 -> [_]
          tunnel: [w167] -> w155 mode=indexing
          i -> [w184]
          n186 = local read "VIRef"() -> (w187:refnum<vi>[])
          n187 = Index Array(array=w187, index=w184) -> (element=w175:refnum<vi>)
          n188 = invoke class="VI" method="Ctrl Val.Get"(reference=w175, "Control Name"="SetVoltageStr") -> (reference out=w169:refnum<vi>, error out=w182:errorcluster, "Get Control Value Variant"=w186:variant)  [unwired: 2 in, 1 out]
          n189 = Variant To Data(error in=w182, type="" ("Control Name"), Variant=w186) -> (data=w181:string, error out=w180:errorcluster)
          n190 = Scan From String(format string="%f", input string=w181, error in=w180) -> (error out=w168:errorcluster, output 1=w166:dbl)  [unwired: 2 in, 2 out]
          n191 = Multiply(x=w166, y="Comm. voltage %") -> (x*y=w176:dbl)
          n192 = Divide(x=w176, y=100.0) -> (x/y=w178:dbl)
          n193 = local read "Common volt. inc"() -> (w165:bool)
          n194 = local read "Common volt. dec"() -> (w163:bool)
          n195 = case shown="True" w165 {
            tunnel: w178 -> [w192 w196]
            tunnel: w166 -> [w193 w195]
            tunnel: [w193 w194] -> w164
            tunnel: [w192 _] -> w162
            frame False {
            }
            frame True {
              n196 = Add(x=w195, y=w196) -> (x+y=w194:dbl)
            }
          }
          n197 = case shown="False" w163 {
            tunnel: w164 -> [w188 w191]
            tunnel: [w188 w190] -> w161
            tunnel: w162 -> [_ w189]
            frame False {
            }
            frame True {
              n198 = Subtract(x=w191, y=w189) -> (x-y=w190:dbl)
            }
          }
          n199 = invoke class="VI" method="Ctrl Val.Set"(reference=w169, error in=w168, "Control Name"="SetVoltage", "Value"=w161) -> (reference out=w171:refnum<vi>, error out=w170:errorcluster)  [unwired: 1 in, 3 out]
          n200 = invoke class="VI" method="Ctrl Val.Set"(reference=w171, error in=w170, "Control Name"="NeedToSetVoltage", "Value"=TRUE ("ConnectChannel")) -> (error out=w167:errorcluster)  [unwired: 1 in, 4 out]
        }
        n201 = Merge Errors(w155) -> (w154:errorcluster)
        n202 = flat-sequence {
          tunnel: w154 -> [w159]
          tunnel: [w159] -> w153
          frame #0 {
            w158 = FALSE ("ConnectChannel")
            n203 = local write "Common volt. inc"(w158) -> ()
            n204 = local write "Common volt. dec"(w158) -> ()
          }
        }
      }
      event "DisconnectChannel": Value Change {
        n205 = event-data() -> ()  [unwired: 7 out]
        n206 = property on="List of channels" class="MCListbox (strict)"() -> ("Value"=w201:i32)  [unwired: 2 in, 2 out]
        n207 = flat-sequence {
          tunnel: w201 -> [w203]
          tunnel: [w203] -> w200
          tunnel: w200 -> [w205]
          tunnel: [w204] -> w198
          tunnel: [w210] -> w199
          tunnel: w198 -> [w210]
          frame #0 {
            w202 = u8 2 ("Disabled")
            n208 = property on="AddChannel" class="Bool (strict)"("Disabled"=w202) -> ()  [unwired: 2 in, 2 out]
            n209 = property on="Set Output ON All" class="Bool (strict)"("Disabled"=w202) -> ()  [unwired: 2 in, 2 out]
            n210 = property on="CurrentModulationB" class="Bool (strict)"("Disabled"=w202) -> ()  [unwired: 2 in, 2 out]
            n211 = property on="ConnectAll" class="Bool (strict)"("Disabled"=w202) -> ()  [unwired: 2 in, 2 out]
            n212 = property on="DisconnectChannel" class="Bool (strict)"("Disabled"=w202) -> ()  [unwired: 2 in, 2 out]
            n213 = property on="ReadFromFile" class="Bool (strict)"("Disabled"=w202) -> ()  [unwired: 2 in, 2 out]
            n214 = property on="Quit" class="Bool (strict)"("Disabled"=w202) -> ()  [unwired: 2 in, 2 out]
            n215 = property on="ConnectChannel" class="Bool (strict)"("Disabled"=w202) -> ()  [unwired: 2 in, 2 out]
            n216 = property on="DeleteChannel" class="Bool (strict)"("Disabled"=w202) -> ()  [unwired: 2 in, 2 out]
            n217 = property on="WriteToFile" class="Bool (strict)"("Disabled"=w202) -> ()  [unwired: 2 in, 2 out]
            n218 = property on="SetCurrentB" class="Bool (strict)"("Disabled"=w202) -> ()  [unwired: 2 in, 2 out]
            n219 = property on="SetOutputOnB" class="Bool (strict)"("Disabled"=w202) -> ()  [unwired: 2 in, 2 out]
            n220 = property on="SetVoltageB" class="Bool (strict)"("Disabled"=w202) -> ()  [unwired: 2 in, 2 out]
            n221 = property on="SetOutputOffB" class="Bool (strict)"("Disabled"=w202) -> ()  [unwired: 2 in, 2 out]
            n222 = property on="SetVoltageAll" class="Bool (strict)"("Disabled"=w202) -> ()  [unwired: 2 in, 2 out]
            n223 = property on="SetCurrentAll" class="Bool (strict)"("Disabled"=w202) -> ()  [unwired: 2 in, 2 out]
            n224 = property on="DisconnectAll" class="Bool (strict)"("Disabled"=w202) -> ()  [unwired: 2 in, 2 out]
          }
          frame #1 {
            w206 = FALSE ("OK Button")
            n225 = local write "DisconnectChannel"(w206) -> ()
            n226 = local read "VIRef"() -> (w208:refnum<vi>[])
            n227 = Index Array(array=w208, index=w205) -> (element=w207:refnum<vi>)
            n228 = invoke class="VI" method="Ctrl Val.Set"(reference=w207, "Control Name"="Connect", "Value"=w206) -> (error out=w204:errorcluster)  [unwired: 2 in, 4 out]
          }
          frame #2 {
            w211 = u8 0 ("Disabled")
            n229 = property on="AddChannel" class="Bool (strict)"("Disabled"=w211) -> ()  [unwired: 2 in, 2 out]
            n230 = property on="CurrentModulationB" class="Bool (strict)"("Disabled"=w211) -> ()  [unwired: 2 in, 2 out]
            n231 = property on="DisconnectChannel" class="Bool (strict)"("Disabled"=w211) -> ()  [unwired: 2 in, 2 out]
            n232 = property on="ConnectAll" class="Bool (strict)"("Disabled"=w211) -> ()  [unwired: 2 in, 2 out]
            n233 = property on="ReadFromFile" class="Bool (strict)"("Disabled"=w211) -> ()  [unwired: 2 in, 2 out]
            n234 = property on="ConnectChannel" class="Bool (strict)"("Disabled"=w211) -> ()  [unwired: 2 in, 2 out]
            n235 = property on="Quit" class="Bool (strict)"("Disabled"=w211) -> ()  [unwired: 2 in, 2 out]
            n236 = property on="DeleteChannel" class="Bool (strict)"("Disabled"=w211) -> ()  [unwired: 2 in, 2 out]
            n237 = property on="SetOutputOffB" class="Bool (strict)"("Disabled"=w211) -> ()  [unwired: 2 in, 2 out]
            n238 = property on="Set Output ON All" class="Bool (strict)"("Disabled"=w211) -> ()  [unwired: 2 in, 2 out]
            n239 = property on="SetVoltageAll" class="Bool (strict)"("Disabled"=w211) -> ()  [unwired: 2 in, 2 out]
            n240 = property on="SetCurrentAll" class="Bool (strict)"("Disabled"=w211) -> ()  [unwired: 2 in, 2 out]
            n241 = property on="DisconnectAll" class="Bool (strict)"("Disabled"=w211) -> ()  [unwired: 2 in, 2 out]
            n242 = property on="WriteToFile" class="Bool (strict)"("Disabled"=w211) -> ()  [unwired: 2 in, 2 out]
            n243 = property on="SetCurrentB" class="Bool (strict)"("Disabled"=w211) -> ()  [unwired: 2 in, 2 out]
            n244 = property on="SetOutputOnB" class="Bool (strict)"("Disabled"=w211) -> ()  [unwired: 2 in, 2 out]
            n245 = property on="SetVoltageB" class="Bool (strict)"("Disabled"=w211) -> ()  [unwired: 2 in, 2 out]
          }
        }
        n246 = Merge Errors(w199) -> (w197:errorcluster)
      }
      event "ConnectChannel": Value Change {
        n247 = event-data() -> ()  [unwired: 7 out]
        n248 = property on="List of channels" class="MCListbox (strict)"() -> ("Value"=w216:i32)  [unwired: 2 in, 2 out]
        n249 = flat-sequence {
          tunnel: w216 -> [w218]
          tunnel: [w218] -> w215
          tunnel: w215 -> [w223]
          tunnel: [w222] -> w213
          tunnel: [w235] -> w214
          tunnel: w213 -> [w235]
          frame #0 {
            w217 = u8 2 ("Disabled")
            n250 = property on="AddChannel" class="Bool (strict)"("Disabled"=w217) -> ()  [unwired: 2 in, 2 out]
            n251 = property on="Set Output ON All" class="Bool (strict)"("Disabled"=w217) -> ()  [unwired: 2 in, 2 out]
            n252 = property on="CurrentModulationB" class="Bool (strict)"("Disabled"=w217) -> ()  [unwired: 2 in, 2 out]
            n253 = property on="ConnectAll" class="Bool (strict)"("Disabled"=w217) -> ()  [unwired: 2 in, 2 out]
            n254 = property on="DisconnectChannel" class="Bool (strict)"("Disabled"=w217) -> ()  [unwired: 2 in, 2 out]
            n255 = property on="ReadFromFile" class="Bool (strict)"("Disabled"=w217) -> ()  [unwired: 2 in, 2 out]
            n256 = property on="Quit" class="Bool (strict)"("Disabled"=w217) -> ()  [unwired: 2 in, 2 out]
            n257 = property on="ConnectChannel" class="Bool (strict)"("Disabled"=w217) -> ()  [unwired: 2 in, 2 out]
            n258 = property on="DeleteChannel" class="Bool (strict)"("Disabled"=w217) -> ()  [unwired: 2 in, 2 out]
            n259 = property on="WriteToFile" class="Bool (strict)"("Disabled"=w217) -> ()  [unwired: 2 in, 2 out]
            n260 = property on="SetCurrentB" class="Bool (strict)"("Disabled"=w217) -> ()  [unwired: 2 in, 2 out]
            n261 = property on="SetOutputOnB" class="Bool (strict)"("Disabled"=w217) -> ()  [unwired: 2 in, 2 out]
            n262 = property on="SetVoltageB" class="Bool (strict)"("Disabled"=w217) -> ()  [unwired: 2 in, 2 out]
            n263 = property on="SetOutputOffB" class="Bool (strict)"("Disabled"=w217) -> ()  [unwired: 2 in, 2 out]
            n264 = property on="SetVoltageAll" class="Bool (strict)"("Disabled"=w217) -> ()  [unwired: 2 in, 2 out]
            n265 = property on="SetCurrentAll" class="Bool (strict)"("Disabled"=w217) -> ()  [unwired: 2 in, 2 out]
            n266 = property on="DisconnectAll" class="Bool (strict)"("Disabled"=w217) -> ()  [unwired: 2 in, 2 out]
          }
          frame #1 {
            n267 = local read "VIRef"() -> (w224:refnum<vi>[])
            n268 = Index Array(array=w224, index=w223) -> (element=w221:refnum<vi>)
            n269 = flat-sequence {
              tunnel: w221 -> [w226]
              tunnel: [w225] -> w219
              tunnel: [w229] -> w220
              tunnel: w219 -> [w229]
              tunnel: [w231] -> w222
              tunnel: w220 -> [w232]
              frame #0 {
                n270 = invoke class="VI" method="Ctrl Val.Set"(reference=w226, "Control Name"="Connect", "Value"=FALSE ("OK Button")) -> (reference out=w225:refnum<vi>)  [unwired: 2 in, 4 out]
              }
              frame #1 {
                n271 = Wait (ms)(milliseconds to wait=u32 1000) -> ()  [unwired: 1 out]
              }
              frame #2 {
                n272 = invoke class="VI" method="Ctrl Val.Set"(reference=w232, "Control Name"="Connect", "Value"=TRUE ("OK Button")) -> (error out=w231:errorcluster)  [unwired: 2 in, 4 out]
              }
            }
          }
          frame #2 {
            w236 = u8 0 ("Disabled")
            n273 = local write "ConnectChannel"(FALSE ("ConnectChannel")) -> ()
            n274 = property on="ConnectAll" class="Bool (strict)"("Disabled"=w236) -> ()  [unwired: 2 in, 2 out]
            n275 = property on="Set Output ON All" class="Bool (strict)"("Disabled"=w236) -> ()  [unwired: 2 in, 2 out]
            n276 = property on="AddChannel" class="Bool (strict)"("Disabled"=w236) -> ()  [unwired: 2 in, 2 out]
            n277 = property on="DisconnectChannel" class="Bool (strict)"("Disabled"=w236) -> ()  [unwired: 2 in, 2 out]
            n278 = property on="ReadFromFile" class="Bool (strict)"("Disabled"=w236) -> ()  [unwired: 2 in, 2 out]
            n279 = property on="ConnectChannel" class="Bool (strict)"("Disabled"=w236) -> ()  [unwired: 2 in, 2 out]
            n280 = property on="Quit" class="Bool (strict)"("Disabled"=w236) -> ()  [unwired: 2 in, 2 out]
            n281 = property on="DeleteChannel" class="Bool (strict)"("Disabled"=w236) -> ()  [unwired: 2 in, 2 out]
            n282 = property on="WriteToFile" class="Bool (strict)"("Disabled"=w236) -> ()  [unwired: 2 in, 2 out]
            n283 = property on="CurrentModulationB" class="Bool (strict)"("Disabled"=w236) -> ()  [unwired: 2 in, 2 out]
            n284 = property on="SetCurrentB" class="Bool (strict)"("Disabled"=w236) -> ()  [unwired: 2 in, 2 out]
            n285 = property on="SetOutputOnB" class="Bool (strict)"("Disabled"=w236) -> ()  [unwired: 2 in, 2 out]
            n286 = property on="SetVoltageB" class="Bool (strict)"("Disabled"=w236) -> ()  [unwired: 2 in, 2 out]
            n287 = property on="SetOutputOffB" class="Bool (strict)"("Disabled"=w236) -> ()  [unwired: 2 in, 2 out]
            n288 = property on="SetVoltageAll" class="Bool (strict)"("Disabled"=w236) -> ()  [unwired: 2 in, 2 out]
            n289 = property on="SetCurrentAll" class="Bool (strict)"("Disabled"=w236) -> ()  [unwired: 2 in, 2 out]
            n290 = property on="DisconnectAll" class="Bool (strict)"("Disabled"=w236) -> ()  [unwired: 2 in, 2 out]
          }
        }
        n291 = Merge Errors(w214) -> (w212:errorcluster)
      }
      event "ConnectAll": Value Change {
        n292 = event-data() -> ()  [unwired: 7 out]
        n293 = flat-sequence {
          tunnel: [w242] -> w239
          tunnel: [w251] -> w240
          tunnel: w239 -> [w251]
          frame #0 {
            w241 = u8 2 ("Disabled")
            n294 = property on="Quit" class="Bool (strict)"("Disabled"=w241) -> ()  [unwired: 2 in, 2 out]
            n295 = property on="ReadFromFile" class="Bool (strict)"("Disabled"=w241) -> ()  [unwired: 2 in, 2 out]
            n296 = property on="CurrentModulationB" class="Bool (strict)"("Disabled"=w241) -> ()  [unwired: 2 in, 2 out]
            n297 = property on="WriteToFile" class="Bool (strict)"("Disabled"=w241) -> ()  [unwired: 2 in, 2 out]
            n298 = property on="ConnectAll" class="Bool (strict)"("Disabled"=w241) -> ()  [unwired: 2 in, 2 out]
            n299 = property on="Set Output ON All" class="Bool (strict)"("Disabled"=w241) -> ()  [unwired: 2 in, 2 out]
            n300 = property on="SetOutputOffB" class="Bool (strict)"("Disabled"=w241) -> ()  [unwired: 2 in, 2 out]
            n301 = property on="AddChannel" class="Bool (strict)"("Disabled"=w241) -> ()  [unwired: 2 in, 2 out]
            n302 = property on="DisconnectChannel" class="Bool (strict)"("Disabled"=w241) -> ()  [unwired: 2 in, 2 out]
            n303 = property on="SetCurrentAll" class="Bool (strict)"("Disabled"=w241) -> ()  [unwired: 2 in, 2 out]
            n304 = property on="SetOutputOnB" class="Bool (strict)"("Disabled"=w241) -> ()  [unwired: 2 in, 2 out]
            n305 = property on="ConnectChannel" class="Bool (strict)"("Disabled"=w241) -> ()  [unwired: 2 in, 2 out]
            n306 = property on="DeleteChannel" class="Bool (strict)"("Disabled"=w241) -> ()  [unwired: 2 in, 2 out]
            n307 = property on="SetCurrentB" class="Bool (strict)"("Disabled"=w241) -> ()  [unwired: 2 in, 2 out]
            n308 = property on="SetVoltageB" class="Bool (strict)"("Disabled"=w241) -> ()  [unwired: 2 in, 2 out]
            n309 = property on="SetVoltageAll" class="Bool (strict)"("Disabled"=w241) -> ()  [unwired: 2 in, 2 out]
            n310 = property on="DisconnectAll" class="Bool (strict)"("Disabled"=w241) -> ()  [unwired: 2 in, 2 out]
          }
          frame #1 {
            n311 = local read "VIRef"() -> (w244:refnum<vi>[])
            n312 = Array Size(array=w244) -> (size(s)=w243:i32)
            n313 = for {
              N: w243 -> [_]
              tunnel: [w245] -> w242 mode=indexing
              i -> [w246]
              n314 = local read "VIRef"() -> (w249:refnum<vi>[])
              n315 = Index Array(array=w249, index=w246) -> (element=w248:refnum<vi>)
              n316 = invoke class="VI" method="Ctrl Val.Set"(reference=w248, "Control Name"="Connect", "Value"=TRUE ("OK Button")) -> (error out=w245:errorcluster)  [unwired: 2 in, 4 out]
            }
          }
          frame #2 {
            w252 = u8 0 ("Disabled")
            n317 = local write "ConnectAll"(FALSE ("ConnectChannel")) -> ()
            n318 = property on="Quit" class="Bool (strict)"("Disabled"=w252) -> ()  [unwired: 2 in, 2 out]
            n319 = property on="AddChannel" class="Bool (strict)"("Disabled"=w252) -> ()  [unwired: 2 in, 2 out]
            n320 = property on="DisconnectChannel" class="Bool (strict)"("Disabled"=w252) -> ()  [unwired: 2 in, 2 out]
            n321 = property on="ConnectAll" class="Bool (strict)"("Disabled"=w252) -> ()  [unwired: 2 in, 2 out]
            n322 = property on="Set Output ON All" class="Bool (strict)"("Disabled"=w252) -> ()  [unwired: 2 in, 2 out]
            n323 = property on="SetOutputOffB" class="Bool (strict)"("Disabled"=w252) -> ()  [unwired: 2 in, 2 out]
            n324 = property on="SetCurrentAll" class="Bool (strict)"("Disabled"=w252) -> ()  [unwired: 2 in, 2 out]
            n325 = property on="ConnectChannel" class="Bool (strict)"("Disabled"=w252) -> ()  [unwired: 2 in, 2 out]
            n326 = property on="SetVoltageAll" class="Bool (strict)"("Disabled"=w252) -> ()  [unwired: 2 in, 2 out]
            n327 = property on="SetOutputOnB" class="Bool (strict)"("Disabled"=w252) -> ()  [unwired: 2 in, 2 out]
            n328 = property on="CurrentModulationB" class="Bool (strict)"("Disabled"=w252) -> ()  [unwired: 2 in, 2 out]
            n329 = property on="DisconnectAll" class="Bool (strict)"("Disabled"=w252) -> ()  [unwired: 2 in, 2 out]
            n330 = property on="ReadFromFile" class="Bool (strict)"("Disabled"=w252) -> ()  [unwired: 2 in, 2 out]
            n331 = property on="WriteToFile" class="Bool (strict)"("Disabled"=w252) -> ()  [unwired: 2 in, 2 out]
            n332 = property on="SetCurrentB" class="Bool (strict)"("Disabled"=w252) -> ()  [unwired: 2 in, 2 out]
            n333 = property on="SetVoltageB" class="Bool (strict)"("Disabled"=w252) -> ()  [unwired: 2 in, 2 out]
            n334 = property on="DeleteChannel" class="Bool (strict)"("Disabled"=w252) -> ()  [unwired: 2 in, 2 out]
          }
        }
        n335 = Merge Errors(w240) -> (w238:errorcluster)
      }
      event "DisconnectAll": Value Change {
        n336 = event-data() -> ()  [unwired: 7 out]
        n337 = flat-sequence {
          tunnel: [w258] -> w256
          tunnel: [w267] -> w255
          tunnel: w256 -> [w267]
          frame #0 {
            w257 = u8 2 ("Disabled")
            n338 = property on="Quit" class="Bool (strict)"("Disabled"=w257) -> ()  [unwired: 2 in, 2 out]
            n339 = property on="ReadFromFile" class="Bool (strict)"("Disabled"=w257) -> ()  [unwired: 2 in, 2 out]
            n340 = property on="CurrentModulationB" class="Bool (strict)"("Disabled"=w257) -> ()  [unwired: 2 in, 2 out]
            n341 = property on="ConnectAll" class="Bool (strict)"("Disabled"=w257) -> ()  [unwired: 2 in, 2 out]
            n342 = property on="ConnectChannel" class="Bool (strict)"("Disabled"=w257) -> ()  [unwired: 2 in, 2 out]
            n343 = property on="AddChannel" class="Bool (strict)"("Disabled"=w257) -> ()  [unwired: 2 in, 2 out]
            n344 = property on="DisconnectChannel" class="Bool (strict)"("Disabled"=w257) -> ()  [unwired: 2 in, 2 out]
            n345 = property on="Set Output ON All" class="Bool (strict)"("Disabled"=w257) -> ()  [unwired: 2 in, 2 out]
            n346 = property on="WriteToFile" class="Bool (strict)"("Disabled"=w257) -> ()  [unwired: 2 in, 2 out]
            n347 = property on="SetOutputOffB" class="Bool (strict)"("Disabled"=w257) -> ()  [unwired: 2 in, 2 out]
            n348 = property on="SetCurrentAll" class="Bool (strict)"("Disabled"=w257) -> ()  [unwired: 2 in, 2 out]
            n349 = property on="SetOutputOnB" class="Bool (strict)"("Disabled"=w257) -> ()  [unwired: 2 in, 2 out]
            n350 = property on="DeleteChannel" class="Bool (strict)"("Disabled"=w257) -> ()  [unwired: 2 in, 2 out]
            n351 = property on="SetCurrentB" class="Bool (strict)"("Disabled"=w257) -> ()  [unwired: 2 in, 2 out]
            n352 = property on="SetVoltageB" class="Bool (strict)"("Disabled"=w257) -> ()  [unwired: 2 in, 2 out]
            n353 = property on="SetVoltageAll" class="Bool (strict)"("Disabled"=w257) -> ()  [unwired: 2 in, 2 out]
            n354 = property on="DisconnectAll" class="Bool (strict)"("Disabled"=w257) -> ()  [unwired: 2 in, 2 out]
          }
          frame #1 {
            n355 = local read "VIRef"() -> (w260:refnum<vi>[])
            n356 = Array Size(array=w260) -> (size(s)=w259:i32)
            n357 = for {
              N: w259 -> [_]
              tunnel: [w261] -> w258 mode=indexing
              i -> [w262]
              n358 = local read "VIRef"() -> (w265:refnum<vi>[])
              n359 = Index Array(array=w265, index=w262) -> (element=w264:refnum<vi>)
              n360 = invoke class="VI" method="Ctrl Val.Set"(reference=w264, "Control Name"="Connect", "Value"=FALSE ("OK Button")) -> (error out=w261:errorcluster)  [unwired: 2 in, 4 out]
            }
          }
          frame #2 {
            w268 = u8 0 ("Disabled")
            n361 = local write "DisconnectAll"(FALSE ("ConnectChannel")) -> ()
            n362 = property on="Quit" class="Bool (strict)"("Disabled"=w268) -> ()  [unwired: 2 in, 2 out]
            n363 = property on="ConnectAll" class="Bool (strict)"("Disabled"=w268) -> ()  [unwired: 2 in, 2 out]
            n364 = property on="ConnectChannel" class="Bool (strict)"("Disabled"=w268) -> ()  [unwired: 2 in, 2 out]
            n365 = property on="AddChannel" class="Bool (strict)"("Disabled"=w268) -> ()  [unwired: 2 in, 2 out]
            n366 = property on="DisconnectChannel" class="Bool (strict)"("Disabled"=w268) -> ()  [unwired: 2 in, 2 out]
            n367 = property on="ReadFromFile" class="Bool (strict)"("Disabled"=w268) -> ()  [unwired: 2 in, 2 out]
            n368 = property on="Set Output ON All" class="Bool (strict)"("Disabled"=w268) -> ()  [unwired: 2 in, 2 out]
            n369 = property on="WriteToFile" class="Bool (strict)"("Disabled"=w268) -> ()  [unwired: 2 in, 2 out]
            n370 = property on="SetOutputOnB" class="Bool (strict)"("Disabled"=w268) -> ()  [unwired: 2 in, 2 out]
            n371 = property on="CurrentModulationB" class="Bool (strict)"("Disabled"=w268) -> ()  [unwired: 2 in, 2 out]
            n372 = property on="SetCurrentB" class="Bool (strict)"("Disabled"=w268) -> ()  [unwired: 2 in, 2 out]
            n373 = property on="SetVoltageB" class="Bool (strict)"("Disabled"=w268) -> ()  [unwired: 2 in, 2 out]
            n374 = property on="SetVoltageAll" class="Bool (strict)"("Disabled"=w268) -> ()  [unwired: 2 in, 2 out]
            n375 = property on="DisconnectAll" class="Bool (strict)"("Disabled"=w268) -> ()  [unwired: 2 in, 2 out]
            n376 = property on="DeleteChannel" class="Bool (strict)"("Disabled"=w268) -> ()  [unwired: 2 in, 2 out]
            n377 = property on="SetOutputOffB" class="Bool (strict)"("Disabled"=w268) -> ()  [unwired: 2 in, 2 out]
            n378 = property on="SetCurrentAll" class="Bool (strict)"("Disabled"=w268) -> ()  [unwired: 2 in, 2 out]
          }
        }
        n379 = Merge Errors(w255) -> (w254:errorcluster)
      }
      event "SetVoltageB": Value Change {
        n380 = event-data() -> ()  [unwired: 7 out]
        n381 = local write "SetVoltageB"(FALSE ("ConnectChannel")) -> ()
        n382 = flat-sequence {
          tunnel: [w276] -> w272
          tunnel: [w285] -> w271
          tunnel: w272 -> [w285]
          frame #0 {
            w274 = u8 2 ("Disabled")
            n383 = property on="Quit" class="Bool (strict)"("Disabled"=w274) -> ()  [unwired: 2 in, 2 out]
            n384 = property on="AddChannel" class="Bool (strict)"("Disabled"=w274) -> ()  [unwired: 2 in, 2 out]
            n385 = property on="Set Output ON All" class="Bool (strict)"("Disabled"=w274) -> ()  [unwired: 2 in, 2 out]
            n386 = property on="CurrentModulationB" class="Bool (strict)"("Disabled"=w274) -> ()  [unwired: 2 in, 2 out]
            n387 = property on="ConnectAll" class="Bool (strict)"("Disabled"=w274) -> ()  [unwired: 2 in, 2 out]
            n388 = property on="DisconnectChannel" class="Bool (strict)"("Disabled"=w274) -> ()  [unwired: 2 in, 2 out]
            n389 = property on="ReadFromFile" class="Bool (strict)"("Disabled"=w274) -> ()  [unwired: 2 in, 2 out]
            n390 = property on="ConnectChannel" class="Bool (strict)"("Disabled"=w274) -> ()  [unwired: 2 in, 2 out]
            n391 = property on="DeleteChannel" class="Bool (strict)"("Disabled"=w274) -> ()  [unwired: 2 in, 2 out]
            n392 = property on="WriteToFile" class="Bool (strict)"("Disabled"=w274) -> ()  [unwired: 2 in, 2 out]
            n393 = property on="SetCurrentB" class="Bool (strict)"("Disabled"=w274) -> ()  [unwired: 2 in, 2 out]
            n394 = property on="SetOutputOnB" class="Bool (strict)"("Disabled"=w274) -> ()  [unwired: 2 in, 2 out]
            n395 = property on="SetVoltageB" class="Bool (strict)"("Disabled"=w274) -> ()  [unwired: 2 in, 2 out]
            n396 = property on="SetOutputOffB" class="Bool (strict)"("Disabled"=w274) -> ()  [unwired: 2 in, 2 out]
            n397 = property on="SetVoltageAll" class="Bool (strict)"("Disabled"=w274) -> ()  [unwired: 2 in, 2 out]
            n398 = property on="SetCurrentAll" class="Bool (strict)"("Disabled"=w274) -> ()  [unwired: 2 in, 2 out]
            n399 = property on="DisconnectAll" class="Bool (strict)"("Disabled"=w274) -> ()  [unwired: 2 in, 2 out]
          }
          frame #1 {
            n400 = property on="List of channels" class="MCListbox (strict)"() -> ("Value"=w275:i32)  [unwired: 2 in, 2 out]
            n401 = local read "VIRef"() -> (w283:refnum<vi>[])
            n402 = local read "SetVoltage"() -> (w281:dbl)
            n403 = Index Array(array=w283, index=w275) -> (element=w282:refnum<vi>)
            n404 = invoke class="VI" method="Ctrl Val.Set"(reference=w282, "Control Name"="SetVoltage", "Value"=w281) -> (reference out=w278:refnum<vi>, error out=w277:errorcluster)  [unwired: 2 in, 3 out]
            n405 = invoke class="VI" method="Ctrl Val.Set"(reference=w278, error in=w277, "Control Name"="NeedToSetVoltage", "Value"=TRUE ("ConnectChannel")) -> (error out=w276:errorcluster)  [unwired: 1 in, 4 out]
          }
          frame #2 {
            w286 = u8 0 ("Disabled")
            n406 = property on="Quit" class="Bool (strict)"("Disabled"=w286) -> ()  [unwired: 2 in, 2 out]
            n407 = property on="ConnectAll" class="Bool (strict)"("Disabled"=w286) -> ()  [unwired: 2 in, 2 out]
            n408 = property on="Set Output ON All" class="Bool (strict)"("Disabled"=w286) -> ()  [unwired: 2 in, 2 out]
            n409 = property on="AddChannel" class="Bool (strict)"("Disabled"=w286) -> ()  [unwired: 2 in, 2 out]
            n410 = property on="CurrentModulationB" class="Bool (strict)"("Disabled"=w286) -> ()  [unwired: 2 in, 2 out]
            n411 = property on="DisconnectChannel" class="Bool (strict)"("Disabled"=w286) -> ()  [unwired: 2 in, 2 out]
            n412 = property on="ReadFromFile" class="Bool (strict)"("Disabled"=w286) -> ()  [unwired: 2 in, 2 out]
            n413 = property on="ConnectChannel" class="Bool (strict)"("Disabled"=w286) -> ()  [unwired: 2 in, 2 out]
            n414 = property on="DeleteChannel" class="Bool (strict)"("Disabled"=w286) -> ()  [unwired: 2 in, 2 out]
            n415 = property on="SetVoltageAll" class="Bool (strict)"("Disabled"=w286) -> ()  [unwired: 2 in, 2 out]
            n416 = property on="SetCurrentAll" class="Bool (strict)"("Disabled"=w286) -> ()  [unwired: 2 in, 2 out]
            n417 = property on="DisconnectAll" class="Bool (strict)"("Disabled"=w286) -> ()  [unwired: 2 in, 2 out]
            n418 = property on="WriteToFile" class="Bool (strict)"("Disabled"=w286) -> ()  [unwired: 2 in, 2 out]
            n419 = property on="SetCurrentB" class="Bool (strict)"("Disabled"=w286) -> ()  [unwired: 2 in, 2 out]
            n420 = property on="SetOutputOnB" class="Bool (strict)"("Disabled"=w286) -> ()  [unwired: 2 in, 2 out]
            n421 = property on="SetVoltageB" class="Bool (strict)"("Disabled"=w286) -> ()  [unwired: 2 in, 2 out]
            n422 = property on="SetOutputOffB" class="Bool (strict)"("Disabled"=w286) -> ()  [unwired: 2 in, 2 out]
          }
        }
        n423 = Merge Errors(w271) -> (w270:errorcluster)
      }
      event "SetOutputOnB": Value Change {
        n424 = event-data() -> ()  [unwired: 2 out]
        n425 = property on="List of channels" class="MCListbox (strict)"() -> ("Value"=w290:i32)  [unwired: 2 in, 2 out]
        n426 = flat-sequence {
          tunnel: w290 -> [w292]
          tunnel: [w292] -> w289
          tunnel: w289 -> [w299]
          tunnel: [w294] -> w288
          tunnel: [w304] -> w287
          tunnel: w288 -> [w304]
          frame #0 {
            w291 = u8 2 ("Disabled")
            n427 = property on="ConnectAll" class="Bool (strict)"("Disabled"=w291) -> ()  [unwired: 2 in, 2 out]
            n428 = property on="Set Output ON All" class="Bool (strict)"("Disabled"=w291) -> ()  [unwired: 2 in, 2 out]
            n429 = property on="AddChannel" class="Bool (strict)"("Disabled"=w291) -> ()  [unwired: 2 in, 2 out]
            n430 = property on="CurrentModulationB" class="Bool (strict)"("Disabled"=w291) -> ()  [unwired: 2 in, 2 out]
            n431 = property on="DisconnectChannel" class="Bool (strict)"("Disabled"=w291) -> ()  [unwired: 2 in, 2 out]
            n432 = property on="ReadFromFile" class="Bool (strict)"("Disabled"=w291) -> ()  [unwired: 2 in, 2 out]
            n433 = property on="Quit" class="Bool (strict)"("Disabled"=w291) -> ()  [unwired: 2 in, 2 out]
            n434 = property on="ConnectChannel" class="Bool (strict)"("Disabled"=w291) -> ()  [unwired: 2 in, 2 out]
            n435 = property on="DeleteChannel" class="Bool (strict)"("Disabled"=w291) -> ()  [unwired: 2 in, 2 out]
            n436 = property on="WriteToFile" class="Bool (strict)"("Disabled"=w291) -> ()  [unwired: 2 in, 2 out]
            n437 = property on="SetCurrentB" class="Bool (strict)"("Disabled"=w291) -> ()  [unwired: 2 in, 2 out]
            n438 = property on="SetOutputOnB" class="Bool (strict)"("Disabled"=w291) -> ()  [unwired: 2 in, 2 out]
            n439 = property on="SetVoltageB" class="Bool (strict)"("Disabled"=w291) -> ()  [unwired: 2 in, 2 out]
            n440 = property on="SetOutputOffB" class="Bool (strict)"("Disabled"=w291) -> ()  [unwired: 2 in, 2 out]
            n441 = property on="SetVoltageAll" class="Bool (strict)"("Disabled"=w291) -> ()  [unwired: 2 in, 2 out]
            n442 = property on="SetCurrentAll" class="Bool (strict)"("Disabled"=w291) -> ()  [unwired: 2 in, 2 out]
            n443 = property on="DisconnectAll" class="Bool (strict)"("Disabled"=w291) -> ()  [unwired: 2 in, 2 out]
          }
          frame #1 {
            n444 = local read "VIRef"() -> (w302:refnum<vi>[])
            n445 = local write "SetOutputOnB"(FALSE ("ConnectChannel")) -> ()
            n446 = Index Array(array=w302, index=w299) -> (element=w301:refnum<vi>)
            n447 = invoke class="VI" method="Ctrl Val.Set"(reference=w301, "Control Name"="SetOutput", "Value"=TRUE ("ConnectChannel")) -> (reference out=w296:refnum<vi>, error out=w295:errorcluster)  [unwired: 2 in, 3 out]
            n448 = invoke class="VI" method="Ctrl Val.Set"(reference=w296, error in=w295, "Control Name"="NeedToSetOutput", "Value"=TRUE ("ConnectChannel")) -> (error out=w294:errorcluster)  [unwired: 1 in, 4 out]
          }
          frame #2 {
            w305 = u8 0 ("Disabled")
            n449 = property on="ConnectAll" class="Bool (strict)"("Disabled"=w305) -> ()  [unwired: 2 in, 2 out]
            n450 = property on="Set Output ON All" class="Bool (strict)"("Disabled"=w305) -> ()  [unwired: 2 in, 2 out]
            n451 = property on="AddChannel" class="Bool (strict)"("Disabled"=w305) -> ()  [unwired: 2 in, 2 out]
            n452 = property on="DisconnectChannel" class="Bool (strict)"("Disabled"=w305) -> ()  [unwired: 2 in, 2 out]
            n453 = property on="ReadFromFile" class="Bool (strict)"("Disabled"=w305) -> ()  [unwired: 2 in, 2 out]
            n454 = property on="ConnectChannel" class="Bool (strict)"("Disabled"=w305) -> ()  [unwired: 2 in, 2 out]
            n455 = property on="Quit" class="Bool (strict)"("Disabled"=w305) -> ()  [unwired: 2 in, 2 out]
            n456 = property on="DeleteChannel" class="Bool (strict)"("Disabled"=w305) -> ()  [unwired: 2 in, 2 out]
            n457 = property on="SetOutputOffB" class="Bool (strict)"("Disabled"=w305) -> ()  [unwired: 2 in, 2 out]
            n458 = property on="CurrentModulationB" class="Bool (strict)"("Disabled"=w305) -> ()  [unwired: 2 in, 2 out]
            n459 = property on="SetVoltageAll" class="Bool (strict)"("Disabled"=w305) -> ()  [unwired: 2 in, 2 out]
            n460 = property on="SetCurrentAll" class="Bool (strict)"("Disabled"=w305) -> ()  [unwired: 2 in, 2 out]
            n461 = property on="DisconnectAll" class="Bool (strict)"("Disabled"=w305) -> ()  [unwired: 2 in, 2 out]
            n462 = property on="WriteToFile" class="Bool (strict)"("Disabled"=w305) -> ()  [unwired: 2 in, 2 out]
            n463 = property on="SetCurrentB" class="Bool (strict)"("Disabled"=w305) -> ()  [unwired: 2 in, 2 out]
            n464 = property on="SetOutputOnB" class="Bool (strict)"("Disabled"=w305) -> ()  [unwired: 2 in, 2 out]
            n465 = property on="SetVoltageB" class="Bool (strict)"("Disabled"=w305) -> ()  [unwired: 2 in, 2 out]
          }
        }
      }
      event "Set Output ON All": Value Change {
        n466 = event-data() -> ("NewVal"=w306:bool)  [unwired: 1 out]
        n467 = flat-sequence {
          tunnel: [w311] -> w307
          tunnel: w306 -> [w311]
          tunnel: [w316] -> w309
          tunnel: w307 -> [w313]
          tunnel: [w327] -> w310
          tunnel: w309 -> [w327]
          frame #0 {
            w312 = u8 2 ("Disabled")
            n468 = property on="Quit" class="Bool (strict)"("Disabled"=w312) -> ()  [unwired: 2 in, 2 out]
            n469 = property on="AddChannel" class="Bool (strict)"("Disabled"=w312) -> ()  [unwired: 2 in, 2 out]
            n470 = property on="CurrentModulationB" class="Bool (strict)"("Disabled"=w312) -> ()  [unwired: 2 in, 2 out]
            n471 = property on="DisconnectChannel" class="Bool (strict)"("Disabled"=w312) -> ()  [unwired: 2 in, 2 out]
            n472 = property on="ConnectAll" class="Bool (strict)"("Disabled"=w312) -> ()  [unwired: 2 in, 2 out]
            n473 = property on="ReadFromFile" class="Bool (strict)"("Disabled"=w312) -> ()  [unwired: 2 in, 2 out]
            n474 = property on="ConnectChannel" class="Bool (strict)"("Disabled"=w312) -> ()  [unwired: 2 in, 2 out]
            n475 = property on="DeleteChannel" class="Bool (strict)"("Disabled"=w312) -> ()  [unwired: 2 in, 2 out]
            n476 = property on="WriteToFile" class="Bool (strict)"("Disabled"=w312) -> ()  [unwired: 2 in, 2 out]
            n477 = property on="SetCurrentB" class="Bool (strict)"("Disabled"=w312) -> ()  [unwired: 2 in, 2 out]
            n478 = property on="SetOutputOnB" class="Bool (strict)"("Disabled"=w312) -> ()  [unwired: 2 in, 2 out]
            n479 = property on="SetVoltageB" class="Bool (strict)"("Disabled"=w312) -> ()  [unwired: 2 in, 2 out]
            n480 = property on="SetOutputOffB" class="Bool (strict)"("Disabled"=w312) -> ()  [unwired: 2 in, 2 out]
            n481 = property on="SetVoltageAll" class="Bool (strict)"("Disabled"=w312) -> ()  [unwired: 2 in, 2 out]
            n482 = property on="SetCurrentAll" class="Bool (strict)"("Disabled"=w312) -> ()  [unwired: 2 in, 2 out]
            n483 = property on="DisconnectAll" class="Bool (strict)"("Disabled"=w312) -> ()  [unwired: 2 in, 2 out]
          }
          frame #1 {
            n484 = local read "VIRef"() -> (w315:refnum<vi>[])
            n485 = Array Size(array=w315) -> (size(s)=w314:i32)
            n486 = for {
              N: w314 -> [_]
              tunnel: [w318] -> w316 mode=indexing
              tunnel: w313 -> [w317]
              i -> [w320]
              n487 = local read "VIRef"() -> (w325:refnum<vi>[])
              n488 = Index Array(array=w325, index=w320) -> (element=w324:refnum<vi>)
              n489 = invoke class="VI" method="Ctrl Val.Set"(reference=w324, "Control Name"="SetOutput", "Value"=w317) -> (reference out=w321:refnum<vi>, error out=w319:errorcluster)  [unwired: 2 in, 3 out]
              n490 = invoke class="VI" method="Ctrl Val.Set"(reference=w321, error in=w319, "Control Name"="NeedToSetOutput", "Value"=TRUE ("ConnectChannel")) -> (error out=w318:errorcluster)  [unwired: 1 in, 4 out]
            }
          }
          frame #2 {
            w328 = u8 0 ("Disabled")
            n491 = disable-structure shown="Disabled" {
              frame Disabled {
                n492 = local write "Set Output ON All"(FALSE ("ConnectChannel")) -> ()
              }
              frame Enabled {
              }
            }
            n493 = property on="Quit" class="Bool (strict)"("Disabled"=w328) -> ()  [unwired: 2 in, 2 out]
            n494 = property on="ConnectAll" class="Bool (strict)"("Disabled"=w328) -> ()  [unwired: 2 in, 2 out]
            n495 = property on="Set Output ON All" class="Bool (strict)"("Disabled"=w328) -> ()  [unwired: 2 in, 2 out]
            n496 = property on="AddChannel" class="Bool (strict)"("Disabled"=w328) -> ()  [unwired: 2 in, 2 out]
            n497 = property on="DisconnectChannel" class="Bool (strict)"("Disabled"=w328) -> ()  [unwired: 2 in, 2 out]
            n498 = property on="ReadFromFile" class="Bool (strict)"("Disabled"=w328) -> ()  [unwired: 2 in, 2 out]
            n499 = property on="ConnectChannel" class="Bool (strict)"("Disabled"=w328) -> ()  [unwired: 2 in, 2 out]
            n500 = property on="DeleteChannel" class="Bool (strict)"("Disabled"=w328) -> ()  [unwired: 2 in, 2 out]
            n501 = property on="SetVoltageB" class="Bool (strict)"("Disabled"=w328) -> ()  [unwired: 2 in, 2 out]
            n502 = property on="CurrentModulationB" class="Bool (strict)"("Disabled"=w328) -> ()  [unwired: 2 in, 2 out]
            n503 = property on="SetOutputOffB" class="Bool (strict)"("Disabled"=w328) -> ()  [unwired: 2 in, 2 out]
            n504 = property on="SetVoltageAll" class="Bool (strict)"("Disabled"=w328) -> ()  [unwired: 2 in, 2 out]
            n505 = property on="SetCurrentAll" class="Bool (strict)"("Disabled"=w328) -> ()  [unwired: 2 in, 2 out]
            n506 = property on="DisconnectAll" class="Bool (strict)"("Disabled"=w328) -> ()  [unwired: 2 in, 2 out]
            n507 = property on="WriteToFile" class="Bool (strict)"("Disabled"=w328) -> ()  [unwired: 2 in, 2 out]
            n508 = property on="SetCurrentB" class="Bool (strict)"("Disabled"=w328) -> ()  [unwired: 2 in, 2 out]
            n509 = property on="SetOutputOnB" class="Bool (strict)"("Disabled"=w328) -> ()  [unwired: 2 in, 2 out]
          }
        }
        n510 = Merge Errors(w310) -> (w308:errorcluster)
      }
      event "SetOutputOffB": Value Change {
        n511 = event-data() -> ()  [unwired: 7 out]
        n512 = local write "SetOutputOffB"(FALSE ("ConnectChannel")) -> ()
        n513 = property on="List of channels" class="MCListbox (strict)"() -> ("Value"=w334:i32)  [unwired: 2 in, 2 out]
        n514 = flat-sequence {
          tunnel: w334 -> [w336]
          tunnel: [w336] -> w333
          tunnel: w333 -> [w343]
          tunnel: [w337] -> w330
          tunnel: [w347] -> w331
          tunnel: w330 -> [w347]
          frame #0 {
            w335 = u8 2 ("Disabled")
            n515 = property on="ConnectAll" class="Bool (strict)"("Disabled"=w335) -> ()  [unwired: 2 in, 2 out]
            n516 = property on="Set Output ON All" class="Bool (strict)"("Disabled"=w335) -> ()  [unwired: 2 in, 2 out]
            n517 = property on="AddChannel" class="Bool (strict)"("Disabled"=w335) -> ()  [unwired: 2 in, 2 out]
            n518 = property on="CurrentModulationB" class="Bool (strict)"("Disabled"=w335) -> ()  [unwired: 2 in, 2 out]
            n519 = property on="DisconnectChannel" class="Bool (strict)"("Disabled"=w335) -> ()  [unwired: 2 in, 2 out]
            n520 = property on="ReadFromFile" class="Bool (strict)"("Disabled"=w335) -> ()  [unwired: 2 in, 2 out]
            n521 = property on="Quit" class="Bool (strict)"("Disabled"=w335) -> ()  [unwired: 2 in, 2 out]
            n522 = property on="ConnectChannel" class="Bool (strict)"("Disabled"=w335) -> ()  [unwired: 2 in, 2 out]
            n523 = property on="DeleteChannel" class="Bool (strict)"("Disabled"=w335) -> ()  [unwired: 2 in, 2 out]
            n524 = property on="WriteToFile" class="Bool (strict)"("Disabled"=w335) -> ()  [unwired: 2 in, 2 out]
            n525 = property on="SetCurrentB" class="Bool (strict)"("Disabled"=w335) -> ()  [unwired: 2 in, 2 out]
            n526 = property on="SetOutputOnB" class="Bool (strict)"("Disabled"=w335) -> ()  [unwired: 2 in, 2 out]
            n527 = property on="SetVoltageB" class="Bool (strict)"("Disabled"=w335) -> ()  [unwired: 2 in, 2 out]
            n528 = property on="SetOutputOffB" class="Bool (strict)"("Disabled"=w335) -> ()  [unwired: 2 in, 2 out]
            n529 = property on="SetVoltageAll" class="Bool (strict)"("Disabled"=w335) -> ()  [unwired: 2 in, 2 out]
            n530 = property on="SetCurrentAll" class="Bool (strict)"("Disabled"=w335) -> ()  [unwired: 2 in, 2 out]
            n531 = property on="DisconnectAll" class="Bool (strict)"("Disabled"=w335) -> ()  [unwired: 2 in, 2 out]
          }
          frame #1 {
            n532 = local read "VIRef"() -> (w345:refnum<vi>[])
            n533 = Index Array(array=w345, index=w343) -> (element=w344:refnum<vi>)
            n534 = invoke class="VI" method="Ctrl Val.Set"(reference=w344, "Control Name"="SetOutput", "Value"=FALSE ("ConnectChannel")) -> (reference out=w340:refnum<vi>, error out=w338:errorcluster)  [unwired: 2 in, 3 out]
            n535 = invoke class="VI" method="Ctrl Val.Set"(reference=w340, error in=w338, "Control Name"="NeedToSetOutput", "Value"=TRUE ("ConnectChannel")) -> (error out=w337:errorcluster)  [unwired: 1 in, 4 out]
          }
          frame #2 {
            w348 = u8 0 ("Disabled")
            n536 = property on="ConnectAll" class="Bool (strict)"("Disabled"=w348) -> ()  [unwired: 2 in, 2 out]
            n537 = property on="Set Output ON All" class="Bool (strict)"("Disabled"=w348) -> ()  [unwired: 2 in, 2 out]
            n538 = property on="AddChannel" class="Bool (strict)"("Disabled"=w348) -> ()  [unwired: 2 in, 2 out]
            n539 = property on="CurrentModulationB" class="Bool (strict)"("Disabled"=w348) -> ()  [unwired: 2 in, 2 out]
            n540 = property on="DisconnectChannel" class="Bool (strict)"("Disabled"=w348) -> ()  [unwired: 2 in, 2 out]
            n541 = property on="ReadFromFile" class="Bool (strict)"("Disabled"=w348) -> ()  [unwired: 2 in, 2 out]
            n542 = property on="ConnectChannel" class="Bool (strict)"("Disabled"=w348) -> ()  [unwired: 2 in, 2 out]
            n543 = property on="Quit" class="Bool (strict)"("Disabled"=w348) -> ()  [unwired: 2 in, 2 out]
            n544 = property on="DeleteChannel" class="Bool (strict)"("Disabled"=w348) -> ()  [unwired: 2 in, 2 out]
            n545 = property on="SetOutputOffB" class="Bool (strict)"("Disabled"=w348) -> ()  [unwired: 2 in, 2 out]
            n546 = property on="SetVoltageAll" class="Bool (strict)"("Disabled"=w348) -> ()  [unwired: 2 in, 2 out]
            n547 = property on="SetCurrentAll" class="Bool (strict)"("Disabled"=w348) -> ()  [unwired: 2 in, 2 out]
            n548 = property on="DisconnectAll" class="Bool (strict)"("Disabled"=w348) -> ()  [unwired: 2 in, 2 out]
            n549 = property on="WriteToFile" class="Bool (strict)"("Disabled"=w348) -> ()  [unwired: 2 in, 2 out]
            n550 = property on="SetCurrentB" class="Bool (strict)"("Disabled"=w348) -> ()  [unwired: 2 in, 2 out]
            n551 = property on="SetOutputOnB" class="Bool (strict)"("Disabled"=w348) -> ()  [unwired: 2 in, 2 out]
            n552 = property on="SetVoltageB" class="Bool (strict)"("Disabled"=w348) -> ()  [unwired: 2 in, 2 out]
          }
        }
      }
      event "WriteToFile": Value Change {
        n553 = event-data() -> ()  [unwired: 7 out]
        n554 = local read "ADRESS"() -> (w353:string[])
        n555 = Array Size(array=w353) -> (size(s)=w352:i32)
        n556 = flat-sequence {
          tunnel: w352 -> [w362]
          tunnel: [w354] -> w350
          tunnel: [w395] -> w351
          tunnel: w350 -> [w395]
          frame #0 {
            n557 = Number To Decimal String(number=w362) -> (decimal integer string=w357:string)  [unwired: 1 out]
            n558 = Write to Text File(text=w357) -> (refnum out=w356:refnum<file>, cancelled=w355:bool, error out=w358:errorcluster)  [unwired: 1 in, 2 out]
            n559 = Write to Text File(file (use dialog)=w356, text="\nИМЯ  АДРЕС  НАПРЯЖЕНИЕ  ТОК", error in=w358) -> (refnum out=w359:refnum<file>, error out=w360:errorcluster)  [unwired: 2 out]
            n560 = for {
              N: w362 -> [_]
              tunnel: w355 -> [w370]
              tunnel: w360 -> [w365]
              tunnel: w359 -> [w372]
              tunnel: [w363] -> w354 mode=indexing
              i -> [w371]
              w377 = "" ("Control Name")
              w384 = "\t"
              n561 = local read "VIRef"() -> (w382:refnum<vi>[])
              n562 = Index Array(array=w382, index=w371) -> (element=w381:refnum<vi>)
              n563 = invoke class="VI" method="Ctrl Val.Get"(reference=w381, "Control Name"="SetVoltageStr") -> (reference out=w375:refnum<vi>, error out=w367:errorcluster, "Get Control Value Variant"=w383:variant)  [unwired: 2 in, 1 out]
              n564 = invoke class="VI" method="Ctrl Val.Get"(reference=w375, error in=w367, "Control Name"="SetCurrentStr") -> (error out=w366:errorcluster, "Get Control Value Variant"=w378:variant)  [unwired: 1 in, 2 out]
              n565 = local read "ADRESS"() -> (w389:string[])
              n566 = local read "NAME"() -> (w387:string[])
              n567 = Index Array(array=w387, index=w371) -> (element=w385:string)
              n568 = Index Array(array=w389, index=w371) -> (element=w388:string)
              n569 = Variant To Data(type=w377, Variant=w378) -> (data=w374:string, error out=w369:errorcluster)  [unwired: 1 in]
              n570 = Variant To Data(type=w377, Variant=w383) -> (data=w379:string, error out=w368:errorcluster)  [unwired: 1 in]
              n571 = Merge Errors(w366, w369, w368, w365) -> (w364:errorcluster)
              n572 = Concatenate Strings("\r\n", w385, w384, w388, w384, w379, w384, w374) -> (w373:string)
              n573 = case shown="True" w370 {
                tunnel: w372 -> [w392 _]
                tunnel: w373 -> [w393 _]
                tunnel: w364 -> [w391 w394]
                tunnel: [w390 w394] -> w363
                frame False {
                  n574 = Write to Text File(file (use dialog)=w392, text=w393, error in=w391) -> (error out=w390:errorcluster)  [unwired: 3 out]
                }
                frame True {
                }
              }
            }
          }
          frame #1 {
            n575 = local write "WriteToFile"(FALSE ("ConnectChannel")) -> ()
          }
        }
        n576 = Merge Errors(w351) -> (w349:errorcluster)
      }
      event "ReadFromFile": Value Change {
        n577 = event-data() -> ()  [unwired: 2 out]
        n578 = local read "ReadFromFile"() -> (w399:bool)
        n579 = Read from Text File(count=100) -> (text=w403:string[], cancelled=w402:bool, error out=w401:errorcluster)  [unwired: 1 in, 3 out]
        n580 = Not(x=w402) -> (.not. x?=w398:bool)
        n581 = And(x=w399, y=w398) -> (x .and. y?=w397:bool)
        n582 = case shown="True" w397 {
          tunnel: w403 -> [_ w407]
          tunnel: w401 -> [w405 w409]
          tunnel: [w405 w408] -> w400
          frame False {
            n583 = local write "ReadFromFile"(FALSE ("ConnectChannel")) -> ()
          }
          frame True {
            n584 = flat-sequence {
              tunnel: w409 -> [w417]
              tunnel: [w416] -> w411
              tunnel: w411 -> [w426]
              tunnel: [w426] -> w410
              tunnel: w410 -> [_]
              tunnel: [w437] -> w413
              tunnel: w407 -> [w436]
              tunnel: w413 -> [w471]
              tunnel: [w471] -> w412
              frame #0 {
                w415 = u8 2 ("Disabled")
                n585 = local read "VIRef"() -> (w418:refnum<vi>[])
                n586 = property on="Set Output ON All" class="Bool (strict)"("Disabled"=w415) -> ()  [unwired: 2 in, 2 out]
                n587 = property on="CurrentModulationB" class="Bool (strict)"("Disabled"=w415) -> ()  [unwired: 2 in, 2 out]
                n588 = property on="ConnectAll" class="Bool (strict)"("Disabled"=w415) -> ()  [unwired: 2 in, 2 out]
                n589 = property on="ReadFromFile" class="Bool (strict)"("Disabled"=w415) -> ()  [unwired: 2 in, 2 out]
                n590 = property on="ConnectChannel" class="Bool (strict)"("Disabled"=w415) -> ()  [unwired: 2 in, 2 out]
                n591 = property on="DisconnectChannel" class="Bool (strict)"("Disabled"=w415) -> ()  [unwired: 2 in, 2 out]
                n592 = property on="WriteToFile" class="Bool (strict)"("Disabled"=w415) -> ()  [unwired: 2 in, 2 out]
                n593 = property on="AddChannel" class="Bool (strict)"("Disabled"=w415) -> ()  [unwired: 2 in, 2 out]
                n594 = property on="SetOutputOnB" class="Bool (strict)"("Disabled"=w415) -> ()  [unwired: 2 in, 2 out]
                n595 = property on="Quit" class="Bool (strict)"("Disabled"=w415) -> ()  [unwired: 2 in, 2 out]
                n596 = property on="DeleteChannel" class="Bool (strict)"("Disabled"=w415) -> ()  [unwired: 2 in, 2 out]
                n597 = property on="SetCurrentB" class="Bool (strict)"("Disabled"=w415) -> ()  [unwired: 2 in, 2 out]
                n598 = property on="SetOutputOffB" class="Bool (strict)"("Disabled"=w415) -> ()  [unwired: 2 in, 2 out]
                n599 = property on="SetCurrentAll" class="Bool (strict)"("Disabled"=w415) -> ()  [unwired: 2 in, 2 out]
                n600 = property on="SetVoltageB" class="Bool (strict)"("Disabled"=w415) -> ()  [unwired: 2 in, 2 out]
                n601 = property on="SetVoltageAll" class="Bool (strict)"("Disabled"=w415) -> ()  [unwired: 2 in, 2 out]
                n602 = property on="DisconnectAll" class="Bool (strict)"("Disabled"=w415) -> ()  [unwired: 2 in, 2 out]
                n603 = Array Size(array=w418) -> (size(s)=w414:i32)
                n604 = for {
                  N: w414 -> [_]
                  tunnel: w418 -> [w422]
                  tunnel: w417 -> [w420]
                  tunnel: [w419] -> w416 mode=indexing
                  i -> [w423]
                  n605 = Index Array(array=w422, index=w423) -> (element=w421:refnum<vi>)
                  n606 = invoke class="VI" method="Ctrl Val.Set"(reference=w421, error in=w420, "Control Name"="Connect", "Value"=FALSE) -> (error out=w419:errorcluster)  [unwired: 1 in, 4 out]
                }
              }
              frame #1 {
                n607 = Wait (ms)(milliseconds to wait=u32 1000) -> ()  [unwired: 1 out]
              }
              frame #2 {
                n608 = local read "VIRef"() -> (w429:refnum<vi>[])
                n609 = Array Size(array=w429) -> (size(s)=w428:i32)
                n610 = for {
                  N: w428 -> [_]
                  tunnel: w429 -> [w431]
                  i -> [w432]
                  n611 = Index Array(array=w431, index=w432) -> (element=w430:refnum<vi>)
                  n612 = invoke class="VI" method="Abort VI"(reference=w430) -> ()  [unwired: 2 in, 3 out]
                }
              }
              frame #3 {
                w434 = string[] [] ("GlobalInAdress")
                n613 = Wait (ms)(milliseconds to wait=u32 250) -> ()  [unwired: 1 out]
                n614 = local write "NAME"(w434) -> ()
                n615 = local write "ADRESS"(w434) -> ()
                n616 = local write "VIRef"(refnum<vi>[] []) -> ()
              }
              frame #4 {
                n617 = Index Array(array=w436, index=0) -> (element=w440:string)
                n618 = Decimal String To Number(string=w440) -> (number=w438:i32)  [unwired: 3 out]
                n619 = for {
                  N: w438 -> [_]
                  tunnel: w436 -> [w465]
                  tunnel: [w441] -> w437 mode=indexing
                  i -> [w468]
                  n620 = Add(x=2, y=w468) -> (x+y=w467:i32)
                  n621 = Index Array(array=w465, index=w467) -> (element=w464:string)
                  n622 = Spreadsheet String To Array(format string="%s", spreadsheet string=w464, array type (2D Dbl)=string[] [] ("GlobalInAdress")) -> (array=w455:string[])  [unwired: 1 out]
                  n623 = Index Array(array=w455, index=3) -> (element=w453:string)
                  n624 = Index Array(array=w455, index=0) -> (element=w459:string)
                  n625 = Index Array(array=w455, index=1) -> (element=w460:string)
                  n626 = Index Array(array=w455, index=2) -> (element=w454:string)
                  n627 = local read "ADRESS"() -> (w451:string[])
                  n628 = Scan From String(input string=w453, default 1=0.0 ("default value 1")) -> (output 1=w446:dbl)  [unwired: 3 in, 3 out]
                  n629 = Scan From String(input string=w454, default 1=0.0 ("default value 1")) -> (output 1=w448:dbl)  [unwired: 3 in, 3 out]
                  n630 = local read "NAME"() -> (w452:string[])
                  n631 = local read "VIRef"() -> (w450:refnum<vi>[])
                  n632 = call "AddChannel.vi"("VIRef"=w450, "Name"=w459, "SetCurrent"=w446, "ADRESS"=w451, "NAME"=w452, "Address"=w460, "SetVoltage"=w448) -> ("NAMEOut"=w445:string[], "error out"=w442:errorcluster, "ADRESSOut"=w443:string[], "VIRefOut"=w444:refnum<vi>[])  [unwired: 1 in, 4 out]
                  n633 = local write "NAME"(w445) -> ()
                  n634 = local write "VIRef"(w444) -> ()
                  n635 = flat-sequence {
                    tunnel: w442 -> [w470]
                    tunnel: [w470] -> w441
                    frame #0 {
                      n636 = Wait (ms)(milliseconds to wait=u32 50) -> ()  [unwired: 1 out]
                    }
                  }
                  n637 = local write "ADRESS"(w443) -> ()
                }
              }
              frame #5 {
                w472 = u8 0 ("Disabled")
                n638 = local write "ReadFromFile"(FALSE ("ConnectChannel")) -> ()
                n639 = property on="ConnectAll" class="Bool (strict)"("Disabled"=w472) -> ()  [unwired: 2 in, 2 out]
                n640 = property on="Set Output ON All" class="Bool (strict)"("Disabled"=w472) -> ()  [unwired: 2 in, 2 out]
                n641 = property on="AddChannel" class="Bool (strict)"("Disabled"=w472) -> ()  [unwired: 2 in, 2 out]
                n642 = property on="CurrentModulationB" class="Bool (strict)"("Disabled"=w472) -> ()  [unwired: 2 in, 2 out]
                n643 = property on="DisconnectChannel" class="Bool (strict)"("Disabled"=w472) -> ()  [unwired: 2 in, 2 out]
                n644 = property on="ReadFromFile" class="Bool (strict)"("Disabled"=w472) -> ()  [unwired: 2 in, 2 out]
                n645 = property on="ConnectChannel" class="Bool (strict)"("Disabled"=w472) -> ()  [unwired: 2 in, 2 out]
                n646 = property on="DeleteChannel" class="Bool (strict)"("Disabled"=w472) -> ()  [unwired: 2 in, 2 out]
                n647 = property on="WriteToFile" class="Bool (strict)"("Disabled"=w472) -> ()  [unwired: 2 in, 2 out]
                n648 = property on="SetCurrentB" class="Bool (strict)"("Disabled"=w472) -> ()  [unwired: 2 in, 2 out]
                n649 = property on="Quit" class="Bool (strict)"("Disabled"=w472) -> ()  [unwired: 2 in, 2 out]
                n650 = property on="SetOutputOnB" class="Bool (strict)"("Disabled"=w472) -> ()  [unwired: 2 in, 2 out]
                n651 = property on="SetVoltageB" class="Bool (strict)"("Disabled"=w472) -> ()  [unwired: 2 in, 2 out]
                n652 = property on="SetOutputOffB" class="Bool (strict)"("Disabled"=w472) -> ()  [unwired: 2 in, 2 out]
                n653 = property on="SetVoltageAll" class="Bool (strict)"("Disabled"=w472) -> ()  [unwired: 2 in, 2 out]
                n654 = property on="SetCurrentAll" class="Bool (strict)"("Disabled"=w472) -> ()  [unwired: 2 in, 2 out]
                n655 = property on="DisconnectAll" class="Bool (strict)"("Disabled"=w472) -> ()  [unwired: 2 in, 2 out]
              }
            }
            n656 = Merge Errors(w412) -> (w408:errorcluster)
          }
        }
      }
      event "SetCurrentB": Value Change {
        n657 = event-data() -> ()  [unwired: 7 out]
        n658 = local write "SetCurrentB"(FALSE ("ConnectChannel")) -> ()
        n659 = property on="List of channels" class="MCListbox (strict)"() -> (error out=w476:errorcluster, "Value"=w480:i32)  [unwired: 2 in, 1 out]
        n660 = flat-sequence {
          tunnel: w480 -> [w483]
          tunnel: [w483] -> w479
          tunnel: [w481] -> w477
          tunnel: w476 -> [w481]
          tunnel: w479 -> [w485]
          tunnel: w477 -> [w484]
          tunnel: [w486] -> w475
          tunnel: [w495] -> w474
          tunnel: w475 -> [w495]
          frame #0 {
            w482 = u8 2 ("Disabled")
            n661 = property on="AddChannel" class="Bool (strict)"("Disabled"=w482) -> ()  [unwired: 2 in, 2 out]
            n662 = property on="Set Output ON All" class="Bool (strict)"("Disabled"=w482) -> ()  [unwired: 2 in, 2 out]
            n663 = property on="CurrentModulationB" class="Bool (strict)"("Disabled"=w482) -> ()  [unwired: 2 in, 2 out]
            n664 = property on="ConnectAll" class="Bool (strict)"("Disabled"=w482) -> ()  [unwired: 2 in, 2 out]
            n665 = property on="DisconnectChannel" class="Bool (strict)"("Disabled"=w482) -> ()  [unwired: 2 in, 2 out]
            n666 = property on="ReadFromFile" class="Bool (strict)"("Disabled"=w482) -> ()  [unwired: 2 in, 2 out]
            n667 = property on="Quit" class="Bool (strict)"("Disabled"=w482) -> ()  [unwired: 2 in, 2 out]
            n668 = property on="ConnectChannel" class="Bool (strict)"("Disabled"=w482) -> ()  [unwired: 2 in, 2 out]
            n669 = property on="DeleteChannel" class="Bool (strict)"("Disabled"=w482) -> ()  [unwired: 2 in, 2 out]
            n670 = property on="WriteToFile" class="Bool (strict)"("Disabled"=w482) -> ()  [unwired: 2 in, 2 out]
            n671 = property on="SetCurrentB" class="Bool (strict)"("Disabled"=w482) -> ()  [unwired: 2 in, 2 out]
            n672 = property on="SetOutputOnB" class="Bool (strict)"("Disabled"=w482) -> ()  [unwired: 2 in, 2 out]
            n673 = property on="SetVoltageB" class="Bool (strict)"("Disabled"=w482) -> ()  [unwired: 2 in, 2 out]
            n674 = property on="SetOutputOffB" class="Bool (strict)"("Disabled"=w482) -> ()  [unwired: 2 in, 2 out]
            n675 = property on="SetVoltageAll" class="Bool (strict)"("Disabled"=w482) -> ()  [unwired: 2 in, 2 out]
            n676 = property on="SetCurrentAll" class="Bool (strict)"("Disabled"=w482) -> ()  [unwired: 2 in, 2 out]
            n677 = property on="DisconnectAll" class="Bool (strict)"("Disabled"=w482) -> ()  [unwired: 2 in, 2 out]
          }
          frame #1 {
            n678 = local read "VIRef"() -> (w493:refnum<vi>[])
            n679 = local read "SetCurrent"() -> (w491:dbl)
            n680 = Index Array(array=w493, index=w485) -> (element=w492:refnum<vi>)
            n681 = invoke class="VI" method="Ctrl Val.Set"(reference=w492, error in=w484, "Control Name"="SetCurrent", "Value"=w491) -> (reference out=w488:refnum<vi>, error out=w487:errorcluster)  [unwired: 1 in, 3 out]
            n682 = invoke class="VI" method="Ctrl Val.Set"(reference=w488, error in=w487, "Control Name"="NeedToSetCurrent", "Value"=TRUE ("ConnectChannel")) -> (error out=w486:errorcluster)  [unwired: 1 in, 4 out]
          }
          frame #2 {
            w496 = u8 0 ("Disabled")
            n683 = property on="AddChannel" class="Bool (strict)"("Disabled"=w496) -> ()  [unwired: 2 in, 2 out]
            n684 = property on="Set Output ON All" class="Bool (strict)"("Disabled"=w496) -> ()  [unwired: 2 in, 2 out]
            n685 = property on="DisconnectChannel" class="Bool (strict)"("Disabled"=w496) -> ()  [unwired: 2 in, 2 out]
            n686 = property on="ConnectAll" class="Bool (strict)"("Disabled"=w496) -> ()  [unwired: 2 in, 2 out]
            n687 = property on="ReadFromFile" class="Bool (strict)"("Disabled"=w496) -> ()  [unwired: 2 in, 2 out]
            n688 = property on="ConnectChannel" class="Bool (strict)"("Disabled"=w496) -> ()  [unwired: 2 in, 2 out]
            n689 = property on="DeleteChannel" class="Bool (strict)"("Disabled"=w496) -> ()  [unwired: 2 in, 2 out]
            n690 = property on="Quit" class="Bool (strict)"("Disabled"=w496) -> ()  [unwired: 2 in, 2 out]
            n691 = property on="WriteToFile" class="Bool (strict)"("Disabled"=w496) -> ()  [unwired: 2 in, 2 out]
            n692 = property on="CurrentModulationB" class="Bool (strict)"("Disabled"=w496) -> ()  [unwired: 2 in, 2 out]
            n693 = property on="SetCurrentB" class="Bool (strict)"("Disabled"=w496) -> ()  [unwired: 2 in, 2 out]
            n694 = property on="SetOutputOnB" class="Bool (strict)"("Disabled"=w496) -> ()  [unwired: 2 in, 2 out]
            n695 = property on="SetVoltageB" class="Bool (strict)"("Disabled"=w496) -> ()  [unwired: 2 in, 2 out]
            n696 = property on="SetOutputOffB" class="Bool (strict)"("Disabled"=w496) -> ()  [unwired: 2 in, 2 out]
            n697 = property on="SetVoltageAll" class="Bool (strict)"("Disabled"=w496) -> ()  [unwired: 2 in, 2 out]
            n698 = property on="SetCurrentAll" class="Bool (strict)"("Disabled"=w496) -> ()  [unwired: 2 in, 2 out]
            n699 = property on="DisconnectAll" class="Bool (strict)"("Disabled"=w496) -> ()  [unwired: 2 in, 2 out]
          }
        }
      }
      event "DeleteChannel": Value Change {
        n700 = event-data() -> ()  [unwired: 7 out]
        n701 = property on="List of channels" class="MCListbox (strict)"() -> ("Value"=w500:i32)  [unwired: 2 in, 2 out]
        n702 = flat-sequence {
          tunnel: [w509] -> w501
          tunnel: w500 -> [w509]
          tunnel: [w513] -> w508
          tunnel: [w511] -> w507
          tunnel: [w512] -> w506
          tunnel: w501 -> [w511]
          tunnel: [w519] -> w505
          tunnel: w508 -> [w519]
          tunnel: [w518] -> w504
          tunnel: w507 -> [w518]
          tunnel: w506 -> [w517]
          tunnel: [w517] -> w503
          tunnel: w505 -> [w524]
          tunnel: [w523] -> w502
          tunnel: w504 -> [w523]
          tunnel: w503 -> [w522]
          tunnel: [w521] -> w498
          tunnel: w502 -> [w526]
          tunnel: [w525] -> w499
          tunnel: w498 -> [w525]
          tunnel: w499 -> [w534]
          tunnel: [w534] -> w497
          frame #0 {
            w510 = u8 2 ("Disabled")
            n703 = property on="AddChannel" class="Bool (strict)"("Disabled"=w510) -> ()  [unwired: 2 in, 2 out]
            n704 = property on="Set Output ON All" class="Bool (strict)"("Disabled"=w510) -> ()  [unwired: 2 in, 2 out]
            n705 = property on="CurrentModulationB" class="Bool (strict)"("Disabled"=w510) -> ()  [unwired: 2 in, 2 out]
            n706 = property on="ConnectAll" class="Bool (strict)"("Disabled"=w510) -> ()  [unwired: 2 in, 2 out]
            n707 = property on="DisconnectChannel" class="Bool (strict)"("Disabled"=w510) -> ()  [unwired: 2 in, 2 out]
            n708 = property on="ReadFromFile" class="Bool (strict)"("Disabled"=w510) -> ()  [unwired: 2 in, 2 out]
            n709 = property on="Quit" class="Bool (strict)"("Disabled"=w510) -> ()  [unwired: 2 in, 2 out]
            n710 = property on="ConnectChannel" class="Bool (strict)"("Disabled"=w510) -> ()  [unwired: 2 in, 2 out]
            n711 = property on="DeleteChannel" class="Bool (strict)"("Disabled"=w510) -> ()  [unwired: 2 in, 2 out]
            n712 = property on="WriteToFile" class="Bool (strict)"("Disabled"=w510) -> ()  [unwired: 2 in, 2 out]
            n713 = property on="SetCurrentB" class="Bool (strict)"("Disabled"=w510) -> ()  [unwired: 2 in, 2 out]
            n714 = property on="SetOutputOnB" class="Bool (strict)"("Disabled"=w510) -> ()  [unwired: 2 in, 2 out]
            n715 = property on="SetVoltageB" class="Bool (strict)"("Disabled"=w510) -> ()  [unwired: 2 in, 2 out]
            n716 = property on="SetOutputOffB" class="Bool (strict)"("Disabled"=w510) -> ()  [unwired: 2 in, 2 out]
            n717 = property on="SetVoltageAll" class="Bool (strict)"("Disabled"=w510) -> ()  [unwired: 2 in, 2 out]
            n718 = property on="SetCurrentAll" class="Bool (strict)"("Disabled"=w510) -> ()  [unwired: 2 in, 2 out]
            n719 = property on="DisconnectAll" class="Bool (strict)"("Disabled"=w510) -> ()  [unwired: 2 in, 2 out]
          }
          frame #1 {
            n720 = local read "VIRef"() -> (w515:refnum<vi>[])
            n721 = Index Array(array=w515, index=w511) -> (element=w513:refnum<vi>)
            n722 = invoke class="VI" method="Ctrl Val.Set"(reference=w513, "Control Name"="Connect", "Value"=FALSE ("OK Button")) -> (error out=w512:errorcluster)  [unwired: 2 in, 4 out]
          }
          frame #2 {
            n723 = Wait (ms)(milliseconds to wait=u32 1000) -> ()  [unwired: 1 out]
          }
          frame #3 {
            n724 = invoke class="VI" method="Abort VI"(reference=w524, error in=w522) -> (error out=w521:errorcluster)  [unwired: 1 in, 2 out]
          }
          frame #4 {
            w527 = 1 ("length")
            n725 = local read "NAME"() -> (w528:string[])
            n726 = local read "VIRef"() -> (w533:refnum<vi>[])
            n727 = Delete From Array(array=w533, length=w527, index=w526) -> (array with subset deleted=w530:refnum<vi>[])  [unwired: 1 out]
            n728 = Delete From Array(array=w528, length=w527, index=w526) -> (array with subset deleted=w529:string[])  [unwired: 1 out]
            n729 = local read "ADRESS"() -> (w532:string[])
            n730 = local write "VIRef"(w530) -> ()
            n731 = local write "NAME"(w529) -> ()
            n732 = Delete From Array(array=w532, length=w527, index=w526) -> (array with subset deleted=w531:string[])  [unwired: 1 out]
            n733 = local write "ADRESS"(w531) -> ()
          }
          frame #5 {
            w535 = u8 0 ("Disabled")
            n734 = local write "DeleteChannel"(FALSE ("DeleteChannel")) -> ()
            n735 = property on="AddChannel" class="Bool (strict)"("Disabled"=w535) -> ()  [unwired: 2 in, 2 out]
            n736 = property on="CurrentModulationB" class="Bool (strict)"("Disabled"=w535) -> ()  [unwired: 2 in, 2 out]
            n737 = property on="DisconnectChannel" class="Bool (strict)"("Disabled"=w535) -> ()  [unwired: 2 in, 2 out]
            n738 = property on="ReadFromFile" class="Bool (strict)"("Disabled"=w535) -> ()  [unwired: 2 in, 2 out]
            n739 = property on="ConnectChannel" class="Bool (strict)"("Disabled"=w535) -> ()  [unwired: 2 in, 2 out]
            n740 = property on="Quit" class="Bool (strict)"("Disabled"=w535) -> ()  [unwired: 2 in, 2 out]
            n741 = property on="DeleteChannel" class="Bool (strict)"("Disabled"=w535) -> ()  [unwired: 2 in, 2 out]
            n742 = property on="WriteToFile" class="Bool (strict)"("Disabled"=w535) -> ()  [unwired: 2 in, 2 out]
            n743 = property on="Set Output ON All" class="Bool (strict)"("Disabled"=w535) -> ()  [unwired: 2 in, 2 out]
            n744 = property on="SetCurrentB" class="Bool (strict)"("Disabled"=w535) -> ()  [unwired: 2 in, 2 out]
            n745 = property on="ConnectAll" class="Bool (strict)"("Disabled"=w535) -> ()  [unwired: 2 in, 2 out]
            n746 = property on="SetOutputOnB" class="Bool (strict)"("Disabled"=w535) -> ()  [unwired: 2 in, 2 out]
            n747 = property on="SetVoltageB" class="Bool (strict)"("Disabled"=w535) -> ()  [unwired: 2 in, 2 out]
            n748 = property on="SetOutputOffB" class="Bool (strict)"("Disabled"=w535) -> ()  [unwired: 2 in, 2 out]
            n749 = property on="SetVoltageAll" class="Bool (strict)"("Disabled"=w535) -> ()  [unwired: 2 in, 2 out]
            n750 = property on="SetCurrentAll" class="Bool (strict)"("Disabled"=w535) -> ()  [unwired: 2 in, 2 out]
            n751 = property on="DisconnectAll" class="Bool (strict)"("Disabled"=w535) -> ()  [unwired: 2 in, 2 out]
          }
        }
      }
    }
    n752 = call <vilib>:"General Error Handler.vi"("type of dialog (OK msg:1)"=u8 0 ("Disabled"), "error in (no error)"=w32) -> ()  [unwired: 14 out]
  }
  n753 = while {
    stop <- FALSE stop-if-true
    n754 = property on="AddChannel" class="Bool (strict)"() -> ("Disabled"=w543:u8)  [unwired: 2 in, 2 out]
    n755 = local read "Quit"() -> (w541:bool)
    n756 = Not(x=w541) -> (.not. x?=w540:bool)
    n757 = Equal?(x=w543, y=u8 0) -> (x = y?=w539:bool)
    n758 = And(x=w540, y=w539) -> (x .and. y?=w538:bool)
    n759 = case shown="True" w538 {
      frame False {
      }
      frame True {
        w545 = string[] [] ("GlobalInAdress")
        n760 = local read "VIRef"() -> (w556:refnum<vi>[])
        n761 = Array Size(array=w556) -> (size(s)=w544:i32)
        n762 = for {
          N: w544 -> [_]
          tunnel: w556 -> [w611]
          shift-right: [w610] -> w553
          shift-left: w545 -> [w609]
          shift-right: [w607] -> w552
          shift-left: w545 -> [w608]
          shift-right: [w598] -> w551
          shift-left: w545 -> [w599]
          shift-right: [w585] -> w550
          shift-left: w545 -> [w594]
          shift-right: [w591] -> w548
          shift-left: w545 -> [w569]
          shift-right: [w583] -> w547
          shift-left: w545 -> [w584]
          i -> [w565]
          w582 = "" ("Control Name")
          n763 = Index Array(array=w611, index=w565) -> (element=w568:refnum<vi>)
          n764 = invoke class="VI" method="Ctrl Val.Get"(reference=w568, "Control Name"="Error") -> (error out=w563:errorcluster, "Get Control Value Variant"=w570:variant)  [unwired: 2 in, 2 out]
          n765 = invoke class="VI" method="Ctrl Val.Get"(reference=w568, "Control Name"="GetCurrent") -> (error out=w579:errorcluster, "Get Control Value Variant"=w604:variant)  [unwired: 2 in, 2 out]
          n766 = invoke class="VI" method="Ctrl Val.Get"(reference=w568, "Control Name"="GetVoltage") -> (error out=w578:errorcluster, "Get Control Value Variant"=w605:variant)  [unwired: 2 in, 2 out]
          n767 = invoke class="VI" method="Ctrl Val.Get"(reference=w568, "Control Name"="SetVoltageStr") -> (error out=w577:errorcluster, "Get Control Value Variant"=w597:variant)  [unwired: 2 in, 2 out]
          n768 = Merge Errors(w563, w579, w578, w577) -> (w573:errorcluster)
          n769 = Variant To Data(type=w582, Variant=w604) -> (data=w601:string)  [unwired: 1 in, 1 out]
          n770 = Variant To Data(type=w582, Variant=w605) -> (data=w602:string)  [unwired: 1 in, 1 out]
          n771 = Variant To Data(type=w582, Variant=w597) -> (data=w589:string)  [unwired: 1 in, 1 out]
          n772 = Variant To Data(type=FALSE, Variant=w570) -> (data=w558:bool)  [unwired: 1 in, 1 out]
          n773 = disable-structure shown="Enabled" {
            disable-tunnel: [w614 w615] -> w559
            disable-tunnel: _ -> [w613 _]
            disable-tunnel: w558 -> [w612 w615]
            frame Disabled {
              n774 = Or(x=w612, y=w613) -> (x .or. y?=w614:bool)
            }
            frame Enabled {
            }
          }
          n775 = Build Array (concatenate)(w608, w601) -> (w607:string[])
          n776 = Build Array (concatenate)(w609, w602) -> (w610:string[])
          n777 = Build Array (concatenate)(w599, w589) -> (w598:string[])
          n778 = invoke class="VI" method="Ctrl Val.Get"(reference=w568, "Control Name"="SetCurrentStr") -> (error out=w576:errorcluster, "Get Control Value Variant"=w596:variant)  [unwired: 2 in, 2 out]
          n779 = invoke class="VI" method="Ctrl Val.Get"(reference=w568, "Control Name"="Output") -> (error out=w575:errorcluster, "Get Control Value Variant"=w586:variant)  [unwired: 2 in, 2 out]
          n780 = invoke class="VI" method="Ctrl Val.Get"(reference=w568, "Control Name"="Active") -> (error out=w574:errorcluster, "Get Control Value Variant"=w593:variant)  [unwired: 2 in, 2 out]
          n781 = Variant To Data(type=w582, Variant=w596) -> (data=w588:string)  [unwired: 1 in, 1 out]
          n782 = Variant To Data "Out"(type=w582, Variant=w586) -> (data=w571:string)  [unwired: 1 in, 1 out]
          n783 = Merge Errors(w576, w575, w574) -> (w572:errorcluster)
          n784 = case shown="True" w559 {
            tunnel: w568 -> [_ w666]
            tunnel: w565 -> [w648 w654]
            tunnel: [w647 w652] -> w560
            frame False {
              n785 = Bundle(w648, "milliseconds to wait"=8) -> (w649:cluster{i32, "milliseconds to wait":i32})  [unwired: 1 in]
              n786 = property on="error" class="MCListbox (strict)"("ActiveCell"=w649, "CellBG"=u32 16777225) -> (error out=w647:errorcluster)  [unwired: 2 in, 1 out]
            }
            frame True {
              w656 = "Connect" ("Control Name")
              n787 = invoke class="VI" method="Ctrl Val.Set"(reference=w666, "Control Name"=w656, "Value"=FALSE ("OK Button")) -> (reference out=w658:refnum<vi>, error out=w661:errorcluster)  [unwired: 2 in, 3 out]
              n788 = flat-sequence {
                tunnel: w661 -> [w671]
                tunnel: [w671] -> w659
                tunnel: w658 -> [w669]
                tunnel: [w669] -> w657
                tunnel: w656 -> [w668]
                tunnel: [w668] -> w655
                tunnel: w654 -> [w667]
                tunnel: [w667] -> w653
                frame #0 {
                  n789 = Wait (ms)(milliseconds to wait=u32 2000) -> ()  [unwired: 1 out]
                }
              }
              n790 = Bundle(w653, "milliseconds to wait"=8) -> (w663:cluster{i32, "milliseconds to wait":i32})  [unwired: 1 in]
              n791 = invoke class="VI" method="Ctrl Val.Set"(reference=w657, error in=w659, "Control Name"=w655, "Value"=TRUE ("OK Button")) -> (error out=w652:errorcluster)  [unwired: 1 in, 4 out]
              n792 = property on="error" class="MCListbox (strict)"("ActiveCell"=w663, "CellBG"=u32 16711680) -> ()  [unwired: 2 in, 2 out]
            }
          }
          n793 = Variant To Data "Active"(type=FALSE, Variant=w593) -> (data=w557:bool)  [unwired: 1 in, 1 out]
          n794 = case shown="\"0\"" w571 {
            tunnel: ["+" ("Control Name") "" ("Control Name") "-" ("Control Name")] -> w562
            tunnel: w565 -> [w616 w621 w626]
            frame "1" {
              n795 = Bundle(w616, "milliseconds to wait"=6) -> (w618:cluster{i32, "milliseconds to wait":i32})  [unwired: 1 in]
              n796 = property on="out" class="MCListbox (strict)"("ActiveCell"=w618, "CellBG"=u32 5895331) -> ()  [unwired: 2 in, 2 out]
            }
            frame Default {
              n797 = Bundle(w621, "milliseconds to wait"=6) -> (w623:cluster{i32, "milliseconds to wait":i32})  [unwired: 1 in]
              n798 = property on="out" class="MCListbox (strict)"("ActiveCell"=w623, "CellBG"=u32 16777225) -> ()  [unwired: 2 in, 2 out]
            }
            frame "0" {
              n799 = Bundle(w626, "milliseconds to wait"=6) -> (w628:cluster{i32, "milliseconds to wait":i32})  [unwired: 1 in]
              n800 = property on="out" class="MCListbox (strict)"("ActiveCell"=w628, "CellBG"=u32 13816530) -> ()  [unwired: 2 in, 2 out]
            }
          }
          n801 = Build Array (concatenate)(w594, w588) -> (w585:string[])
          n802 = case shown="False" w557 {
            tunnel: ["-" ("Control Name") "+" ("Control Name")] -> w592
            tunnel: w565 -> [w633 w642]
            tunnel: w562 -> [_ w641]
            tunnel: ["?" ("Control Name") w641] -> w561
            frame False {
              n803 = Bundle(w633, "milliseconds to wait"=7) -> (w639:cluster{i32, "milliseconds to wait":i32})  [unwired: 1 in]
              n804 = property on="active" class="MCListbox (strict)"("ActiveCell"=w639, "CellBG"=u32 14869218) -> (error out=w634:errorcluster)  [unwired: 2 in, 1 out]
              n805 = Bundle(w633, "milliseconds to wait"=6) -> (w632:cluster{i32, "milliseconds to wait":i32})  [unwired: 1 in]
              n806 = property on="out" class="MCListbox (strict)"(error in=w634, "ActiveCell"=w632, "CellBG"=u32 14869218) -> ()  [unwired: 1 in, 2 out]
            }
            frame True {
              n807 = Bundle(w642, "milliseconds to wait"=7) -> (w644:cluster{i32, "milliseconds to wait":i32})  [unwired: 1 in]
              n808 = property on="active" class="MCListbox (strict)"("ActiveCell"=w644, "CellBG"=u32 5895331) -> ()  [unwired: 2 in, 2 out]
            }
          }
          n809 = Merge Errors(w573, w572, w560) -> (w567:errorcluster)
          n810 = Build Array (concatenate)(w584, w561) -> (w583:string[])
          n811 = Build Array (concatenate)(w569, w592) -> (w591:string[])
          n812 = call <vilib>:"General Error Handler.vi"("type of dialog (OK msg:1)"=u32 0 ("milliseconds to wait"), "error in (no error)"=w567) -> ()  [unwired: 9 in, 5 out]
        }
        n813 = local read "ADRESS"() -> (w554:string[])
        n814 = local read "NAME"() -> (w549:string[])
        n815 = Build Array(w549, w554, w553, w552, w551, w550, w547, w548) -> (w555:string[][])
        n816 = Transpose 2D Array(2D array=w555) -> (transposed array=w546:string[][])
        n817 = property on="List of channels" class="MCListbox (strict)"("ItemNames"=w546) -> ()  [unwired: 2 in, 2 out]
      }
    }
  }
  n818 = property on="Set Output ON All" class="Bool (strict)"("Disabled"=w18) -> (error out=w10:errorcluster)  [unwired: 2 in, 1 out]
  n819 = property on="SetCurrentAll" class="Bool (strict)"("Disabled"=w18) -> ()  [unwired: 2 in, 2 out]
  n820 = property on="AddChannel" class="Bool (strict)"("Disabled"=w18) -> (error out=w17:errorcluster)  [unwired: 2 in, 1 out]
  n821 = property on="AddChannel" class="Bool (strict)"("Disabled"=u8 0) -> ()  [unwired: 2 in, 2 out]
  n822 = property on="IP" class="Str"("Value"="" ("IP")) -> ()  [unwired: 2 in, 2 out]
  n823 = property on="Имя" class="Str"("Value"="" ("Name")) -> ()  [unwired: 2 in, 2 out]
  n824 = local write "WriteToFile"(w21) -> ()
  n825 = local write "DisconnectChannel"(w21) -> ()
  n826 = local write "ConnectChannel"(w21) -> ()
  n827 = local write "SetCurrentB"(w21) -> ()
  n828 = local write "ReadFromFile"(w21) -> ()
  n829 = local write "AddChannel"(w21) -> ()
  n830 = local write "Quit"(w21) -> ()
  n831 = local write "SetCurrentAll"(w21) -> ()
  n832 = local write "SetVoltageAll"(w21) -> ()
  n833 = local write "DeleteChannel"(w21) -> ()
  n834 = local write "SetVoltageB"(w21) -> ()
  n835 = local write "SetOutputOnB"(w20) -> ()
  n836 = local write "ConnectAll"(w20) -> ()
  n837 = local write "SetOutputOffB"(w20) -> ()
  n838 = local write "DisconnectAll"(w20) -> ()
  n839 = local write "CurrentModulationB"(w20) -> ()
  n840 = local write "CurrentModulationOn"(w20) -> ()
  n841 = for "инициализация цветов и размера ячеек табл." {
    N: 50 -> [_]
    i -> [w674]
    n842 = flat-sequence {
      tunnel: w674 -> [w679]
      tunnel: [w679] -> w673
      tunnel: w673 -> [w718]
      tunnel: [w718] -> w672
      tunnel: w672 -> [w731]
      frame #0 {
        w675 = "Application font" ("Font Name")
        n843 = Bundle(w679, 4) -> (w691:cluster{i32, i32})  [unwired: 1 in]
        n844 = property on="active" class="MCListbox (strict)"("ActiveCell"=w691, "Height"=u32 35 ("Active Cell:Cell Size:Height"), "CellFontSize"=u16 28 ("Size")) -> ()  [unwired: 2 in, 2 out]
        n845 = Bundle(w679, 2) -> (w678:cluster{i32, i32})  [unwired: 1 in]
        n846 = Bundle(w679, 3) -> (w692:cluster{i32, i32})  [unwired: 1 in]
        n847 = Bundle(w679, 1) -> (w701:cluster{i32, i32})  [unwired: 1 in]
        n848 = Bundle(w679, 6) -> (w677:cluster{i32, i32})  [unwired: 1 in]
        n849 = Bundle(w679, 5) -> (w676:cluster{i32, i32})  [unwired: 1 in]
        n850 = Bundle(w679, 0) -> (w702:cluster{i32, i32})  [unwired: 1 in]
        n851 = property on="active" class="MCListbox (strict)"("ActiveCell"=w678, "Height"=u32 35 ("Active Cell:Cell Size:Height"), "CellFontSize"=u16 28 ("Size"), "CellFontName"=w675) -> ()  [unwired: 2 in, 2 out]
        n852 = property on="active" class="MCListbox (strict)"("ActiveCell"=w692, "Height"=u32 35 ("Active Cell:Cell Size:Height"), "CellFontSize"=u16 28 ("Size"), "CellFontName"=w675) -> ()  [unwired: 2 in, 2 out]
        n853 = property on="active" class="MCListbox (strict)"("ActiveCell"=w701, "Height"=u32 35 ("Active Cell:Cell Size:Height"), "CellFontSize"=u16 28 ("Size"), "CellFontName"=w675) -> ()  [unwired: 2 in, 2 out]
        n854 = property on="active" class="MCListbox (strict)"("ActiveCell"=w677, "Height"=u32 35 ("Active Cell:Cell Size:Height"), "CellFontSize"=u16 28 ("Size"), "CellFontName"=w675) -> ()  [unwired: 2 in, 2 out]
        n855 = property on="active" class="MCListbox (strict)"("ActiveCell"=w676, "Height"=u32 35 ("Active Cell:Cell Size:Height"), "CellFontSize"=u16 28 ("Size"), "CellFontName"=w675) -> ()  [unwired: 2 in, 2 out]
        n856 = property on="active" class="MCListbox (strict)"("ActiveCell"=w702, "Height"=u32 35 ("Active Cell:Cell Size:Height"), "CellFontSize"=u16 28 ("Size"), "CellFontName"=w675) -> ()  [unwired: 2 in, 2 out]
      }
      frame #1 {
        w714 = T1 {"Font Name"="Application font", "Size"=28, "Bold"=FALSE, "Italic"=FALSE, "Underline"=FALSE, "Strikeout"=FALSE, "Color"=6908265} ("Active Cell:Cell Font")
        w709 = T1 {"Font Name"="Application font", "Size"=30, "Bold"=TRUE, "Italic"=FALSE, "Underline"=FALSE, "Strikeout"=FALSE, "Color"=2263842} ("Active Cell:Cell Font")
        n857 = Bundle(w718, 3) -> (w705:cluster{i32, i32})  [unwired: 1 in]
        n858 = Bundle(w718, 2) -> (w708:cluster{i32, i32})  [unwired: 1 in]
        n859 = Bundle(w718, 0) -> (w716:cluster{i32, i32})  [unwired: 1 in]
        n860 = Bundle(w718, 5) -> (w712:cluster{i32, i32})  [unwired: 1 in]
        n861 = Bundle(w718, 4) -> (w711:cluster{i32, i32})  [unwired: 1 in]
        n862 = property on="active" class="MCListbox (strict)"("ActiveCell"=w705, "CellFont"=w709) -> ()  [unwired: 2 in, 2 out]
        n863 = property on="active" class="MCListbox (strict)"("ActiveCell"=w708, "CellFont"=w709) -> ()  [unwired: 2 in, 2 out]
        n864 = property on="active" class="MCListbox (strict)"("ActiveCell"=w716, "CellFont"=T1 {"Font Name"="Application font", "Size"=28, "Bold"=FALSE, "Italic"=FALSE, "Underline"=FALSE, "Strikeout"=FALSE, "Color"=0} ("Active Cell:Cell Font")) -> ()  [unwired: 2 in, 2 out]
        n865 = property on="active" class="MCListbox (strict)"("ActiveCell"=w712, "CellFont"=w714) -> ()  [unwired: 2 in, 2 out]
        n866 = property on="active" class="MCListbox (strict)"("ActiveCell"=w711, "CellFont"=w714) -> ()  [unwired: 2 in, 2 out]
      }
      frame #2 {
        w730 = T1 {"Font Name"="Application font", "Size"=28, "Bold"=FALSE, "Italic"=FALSE, "Underline"=FALSE, "Strikeout"=FALSE, "Color"=0} ("Active Cell:Cell Font")
        n867 = Bundle(w731, 6) -> (w725:cluster{i32, i32})  [unwired: 1 in]
        n868 = Bundle(w731, 8) -> (w726:cluster{i32, i32})  [unwired: 1 in]
        n869 = Bundle(w731, 7) -> (w727:cluster{i32, i32})  [unwired: 1 in]
        n870 = property on="active" class="MCListbox (strict)"("ActiveCell"=w725, "CellBG"=u32 16777225) -> (error out=w724:errorcluster)  [unwired: 2 in, 1 out]
        n871 = property on="error" class="MCListbox (strict)"("ActiveCell"=w726, "CellBG"=u32 16777225) -> ()  [unwired: 2 in, 2 out]
        n872 = property on="out" class="MCListbox (strict)"("ActiveCell"=w727, "CellBG"=u32 16777225) -> (error out=w728:errorcluster)  [unwired: 2 in, 1 out]
        n873 = property on="active" class="MCListbox (strict)"(error in=w724, "ActiveCell"=w725, "CellFont"=w730) -> ()  [unwired: 1 in, 2 out]
        n874 = property on="active" class="MCListbox (strict)"(error in=w728, "ActiveCell"=w727, "CellFont"=w730) -> ()  [unwired: 1 in, 2 out]
      }
    }
  }
  n875 = property on="CurrentModulationB" class="Bool (strict)"(error in=w17, "Disabled"=w18) -> (error out=w16:errorcluster)  [unwired: 1 in, 1 out]
  n876 = property on="DisconnectAll" class="Bool (strict)"(error in=w10, "Disabled"=w18) -> (error out=w9:errorcluster)  [unwired: 1 in, 1 out]
  n877 = property on="DisconnectChannel" class="Bool (strict)"(error in=w16, "Disabled"=w18) -> (error out=w15:errorcluster)  [unwired: 1 in, 1 out]
  n878 = property on="WriteToFile" class="Bool (strict)"(error in=w9, "Disabled"=w18) -> (error out=w8:errorcluster)  [unwired: 1 in, 1 out]
  n879 = property on="SetCurrentB" class="Bool (strict)"(error in=w8, "Disabled"=w18) -> (error out=w7:errorcluster)  [unwired: 1 in, 1 out]
  n880 = property on="ConnectAll" class="Bool (strict)"(error in=w15, "Disabled"=w18) -> (error out=w14:errorcluster)  [unwired: 1 in, 1 out]
  n881 = property on="Quit" class="Bool (strict)"(error in=w7, "Disabled"=w18) -> (error out=w6:errorcluster)  [unwired: 1 in, 1 out]
  n882 = property on="ReadFromFile" class="Bool (strict)"(error in=w14, "Disabled"=w18) -> (error out=w13:errorcluster)  [unwired: 1 in, 1 out]
  n883 = property on="SetOutputOnB" class="Bool (strict)"(error in=w6, "Disabled"=w18) -> (error out=w5:errorcluster)  [unwired: 1 in, 1 out]
  n884 = property on="ConnectChannel" class="Bool (strict)"(error in=w13, "Disabled"=w18) -> (error out=w12:errorcluster)  [unwired: 1 in, 1 out]
  n885 = property on="SetVoltageB" class="Bool (strict)"(error in=w5, "Disabled"=w18) -> (error out=w4:errorcluster)  [unwired: 1 in, 1 out]
  n886 = property on="SetOutputOffB" class="Bool (strict)"(error in=w4, "Disabled"=w18) -> ()  [unwired: 1 in, 2 out]
  n887 = property on="DeleteChannel" class="Bool (strict)"(error in=w12, "Disabled"=w18) -> (error out=w11:errorcluster)  [unwired: 1 in, 1 out]
  n888 = property on="SetVoltageAll" class="Bool (strict)"(error in=w11, "Disabled"=w18) -> ()  [unwired: 1 in, 2 out]
  "VIRef" <- refnum<vi>[] []
  "ADRESS" <- string[] [] ("GlobalInAdress")
  "NAME" <- string[] [] ("GlobalInAdress")
  "CURRENTSET" <- dbl[] [] ("GlobalInAdress")
